vi "Dashboard custom_bartender&global&gripper&camera2-2.vi"() -> ()   [LabVIEW 2017]
uses:
  C:/Users/IMR Lab/Documents/LabVIEW Data/UniversalRobotsSDK_LABView/LabVIEW/Examples/LabVIEW10/UnderAutomation.UniversalRobots.dll
  UnderAutomation.UniversalRobots.dll
  Global 1.vi
panel:
  out "3rd Order":bool
  out "2nd Order":bool
  out "1st Order":bool
  in  "stop":bool
  out "Rx":dbl
  out "Rz":dbl
  out "Ry":dbl
  out "Enabled":bool
  out "Port":i32
  in  "Move to particular posture":bool
  in  "Move to Zero position":bool
  out "Connected":bool
  in  "Robot IP(192.168.112.182)":string
  out "Connect error":errorcluster
  in  "Power on\nRelease brake":bool
  in  "Power off":bool
  in  "Connect":bool
  in  "Send script":bool
  in  "Script to execute":string
  out "Powered on":bool
  out "X":dbl
  out "Y":dbl
  out "Z":dbl
  out "License state":string
  # "e"
  # "movej( get_inverse_kin(p[0.3138, 0.0814, 0.1647, 0.4226, -2.3876, -2.3851]),  a=0.5, v=0.25, t=0, r=0)"
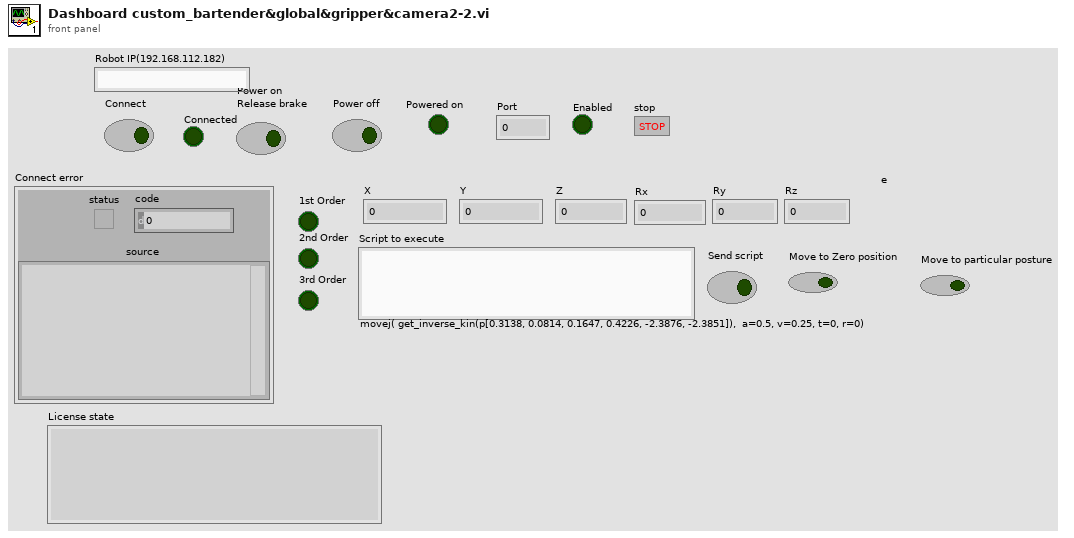
[diagram p1: front panel]
types:
  T1 = enum16{"Standard", "Buffered", "CRLF", "Immediate"}
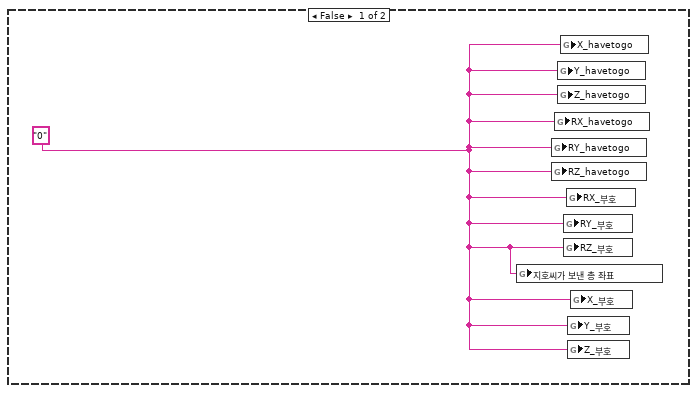
[diagram p2: hidden frame]
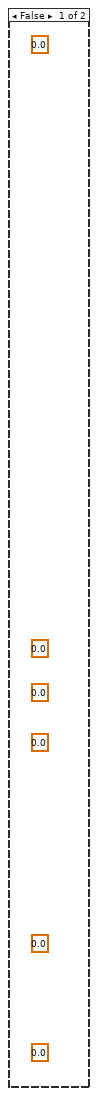
[diagram p3: hidden frame]
diagram:
  w1 = ""
  # "미니콜라 따르는 자세"
  # "술잔 중간지점 가는 자세"
  # "짐빔에서 토닉이동 준비 자세"
  # "술잔 따르는 자세2"
  # "술잔 위로 가는 자세2"
  # "토닉워터 뺴는 자세"
  # "토닉워 들어올리는 자세"
  # "토닉워터 가는 자세"
  # "토닉워터 보는 자세"
  # "짐빔 들어올리는 자세"
  # "짐빔로 가는 자세"
  # "짐빔 보는 자세"
  # "콜라 뺴는 자세"
  # "콜라 들어올리는 자세"
  # "콜라로 가는 자세"
  # "콜라 보는 자세"
  # "술잔 따르는 자세"
  # "술잔 위로 가는 자세"
  # "잭다니엘 들어올리는 자세"
  # "잭다니엘 위치로 가는 자세"
  # "잭다니엘 보는 자세"
  # "1자로 서는 자세"
  # "Example : Display power on status"
  # "Create a UR\ncobot instance"
  # "Show license state"
  # "Register your confidential license key to exit\ntrial period and use this library forever"
  # "Power off when button is clicked"
  # "Power on and release brake when button is clicked"
  # "Get your UR Dashboard interface"
  n1 = global write "Global 1.vi" "TCP 스위치"(FALSE ("TCP 스위치")) -> ()
  n2 = global write "Global 1.vi" "미니콜라 따르는 자세"("movej([-0.0902,-1.8120,-1.9241,-3.5769,6.2827,8.4658], a=0.5, v=0.25, t=0, r=0)") -> ()
  n3 = global write "Global 1.vi" "잭다니엘 들어올리는 자세"("movej([0.8116,-2.0223,-1.2828,-3.0107,4.3284,5.9341], a=0.5, v=0.25, t=0, r=0)") -> ()
  n4 = global write "Global 1.vi" "짐빔 토닉 이동 준비자세"("movej([-0.5421,-0.8131,0.8439,-0.0538,2.5052,5.9032], a=0.5, v=0.25, t=0, r=0)") -> ()
  n5 = global write "Global 1.vi" "토닉 빼는 자세"("movej([-0.5277,-1.5104,1.5889,-0.0548,2.5728,5.9025], a=0.5, v=0.25, t=0, r=0)") -> ()
  n6 = global write "Global 1.vi" "잭다닐 위치로 가는 자세"("movej([0.8116,-2.3119,-1.606,-2.3958,4.3284,5.9341], a=0.5, v=0.25, t=0, r=0)") -> ()
  n7 = global write "Global 1.vi" "토닉 드는 자세"("movej([-1.0311,-1.1460,1.5830,-0.4348,2.0708,5.9048], a=0.5, v=0.25, t=0, r=0)") -> ()
  n8 = global write "Global 1.vi" "토닉 보는 자세"("movej([-0.4690,-1.1292,2.1508,-1.0119,2.6124,5.9032], a=0.5, v=0.25, t=0, r=0)") -> ()
  n9 = global write "Global 1.vi" "술잔 위로 가는 자세 2"("movej([0.0485,-1.6015,2.5780,-1.0382,-0.0520,5.3649], a=0.5, v=0.25, t=0, r=0)") -> ()
  n10 = global write "Global 1.vi" "1자로 서는 자세"("movej([3.1412,-1.5708,0,-1.5708,3.1412,5.8904], a=0.5, v=0.25, t=0, r=0)") -> ()
  n11 = global write "Global 1.vi" "짐빔 들어올리는 자세"("movej([-0.5421,-0.8131,0.8439,-0.0538,2.5052,5.9032], a=0.5, v=0.25, t=0, r=0)") -> ()
  n12 = global write "Global 1.vi" "술잔 위로 가는 자세"("movej([-0.0903,-2.0548,-2.0169,-3.3289,6.2826,7.4091], a=0.5, v=0.25, t=0, r=0)") -> ()
  n13 = global write "Global 1.vi" "토닉 가는자세"("movej([-0.9924,-0.8742,1.7459,-0.8837,2.0958,5.9048], a=0.5, v=0.25, t=0, r=0)") -> ()
  n14 = global write "Global 1.vi" "잭다니엘 보는 자세"("movej([0,-2.2170,-1.4226,-2.2842,3.1412,6.2832], a=0.5, v=0.25, t=0, r=0)") -> ()
  n15 = global write "Global 1.vi" "짐빔 위치로 가는 자세"("movej([-0.5436,-0.4519,0.8428,-0.3534,2.6134,5.9032], a=0.5, v=0.25, t=0, r=0)") -> ()
  n16 = global write "Global 1.vi" "콜라 보는 자세"("movej([0,-1.8110,-2.1684,-2.3033,3.1543,5.9213], a=0.5, v=0.25, t=0, r=0)") -> ()
  n17 = global write "Global 1.vi" "콜라로 가는자세"("movej([1.2020,-2.166,-1.9385,-2.1863,4.3172,5.9210], a=0.5, v=0.25, t=0, r=0)") -> ()
  n18 = global write "Global 1.vi" "콜라 빼는 자세"("movej([0.8789,-1.5237,-2.1070,-2.6679, 3.9917,5.9085], a=0.5, v=0.25, t=0, r=0)") -> ()
  n19 = global write "Global 1.vi" "콜라 드는 자세"("movej([1.2020,-1.8452,-1.7403,-2.7082,4.3162,5.9158], a=0.5, v=0.25, t=0, r=0)") -> ()
  n20 = global write "Global 1.vi" "술 따르는 자세 2"("movej([0.0412,-1.9708,2.4700,-1.0157,-0.0618,4.8998], a=0.5, v=0.25, t=0, r=0)") -> ()
  n21 = global write "Global 1.vi" "잭다니엘 카메라 값"(w1) -> ()
  n22 = global write "Global 1.vi" "술 따르는 자세"("movej([-0.0902,-1.9024,-1.9241,-3.5769,6.2827,8.4692], a=0.5, v=0.25, t=0, r=0)") -> ()
  n23 = global write "Global 1.vi" "짐빔 보는 자세"("movej([-0.0364,-0.6154,0.9421,-0.3291,3.1047,5.9020], a=0.5, v=0.25, t=0, r=0)") -> ()
  n24 = global write "Global 1.vi" "콜라 카메라 값"(w1) -> ()
  n25 = global write "Global 1.vi" "토닉 카메라 값"(w1) -> ()
  n26 = global write "Global 1.vi" "짐빔 카메라 값"(w1) -> ()
  n27 = constructor class="UR"() -> (reference out=w27:refnum<k24>)  [unwired: 3 in, 2 out]
  n28 = global write "Global 1.vi" "술잔 중간지점"("movej([-0.2173,-1.9485,-1.6874,-3.9352,6.2671,7.2276], a=0.5, v=0.25, t=0, r=0)") -> ()
  n29 = while {
    tunnel: w27 -> [w33]
    stop <- FALSE stop-if-true
    # "Connect to the robot when button is pressed"
    # "Show if primary interface is connected"
    # "Get your UR primary interface"
    n30 = property class="UR"(reference=w33) -> ("PrimaryInterface"=w36:refnum<k24>)  [unwired: 1 in, 2 out]
    n31 = Wait (ms)(milliseconds to wait=u32 50) -> ()  [unwired: 1 out]
    n32 = property class="PrimaryInterfaceClientInternal"(reference=w36) -> ("Connected"=w35:bool)  [unwired: 1 in, 2 out]
    "Connected" <- w35
    n33 = case shown="True" "Connect" {
      tunnel: w33 -> [_ w1119]
      frame False {
      }
      frame True {
        n34 = flat-sequence {
          tunnel: w1119 -> [w1121]
          frame #0 {
            n35 = invoke class="UR" method="Connect"(reference=w1121, "ip"="Robot IP(192.168.112.182)") -> (error out=→"Connect error":errorcluster)  [unwired: 2 in, 3 out]
          }
        }
      }
    }
    n36 = case shown="True" w35 {
      tunnel: w36 -> [_ w49]
      frame False {
        (unwired) 0.0 ("Rx")
        (unwired) 0.0 ("Rz")
        (unwired) 0.0 ("Ry")
        (unwired) 0.0 ("Z")
        (unwired) 0.0 ("X")
        (unwired) 0.0 ("Y")
      }
      frame True {
        # "Send URScript when button pressed"
        # "Example : Display current cartesian pose"
        n37 = property class="PrimaryInterfaceClientInternal"(reference=w49) -> ("Script"=w50:refnum<k24>)  [unwired: 1 in, 2 out]
        n38 = global read "Global 1.vi" "2nd Order"() -> (w53:bool)
        "2nd Order" <- w53
        n39 = global read "Global 1.vi" "3rd Order"() -> (w52:bool)
        "3rd Order" <- w52
        n40 = global read "Global 1.vi" "1st Order"() -> (w54:bool)
        "1st Order" <- w54
        n41 = Build Array(w54, w53, w52) -> (w55:bool[])
        n42 = Boolean Array To Number(Boolean array=w55) -> (number=w51:u32)
        n43 = case shown="100" w51 {
          tunnel: w50 -> [_ w106 w433 _ w763 _ _ _]
          frame 0, Default {
          }
          frame 1 {
            # "잭다 : 콜라 = 1 : 3"
            # "1st order"
            n44 = flat-sequence {
              tunnel: w106 -> [w110]
              tunnel: [w109] -> w105
              tunnel: w105 -> [w114]
              tunnel: [w112] -> w99
              tunnel: w99 -> [w117]
              tunnel: [w117] -> w97
              tunnel: w97 -> [w120]
              tunnel: [w120] -> w75
              tunnel: w75 -> [w124]
              tunnel: [w124] -> w72
              tunnel: w72 -> [w131]
              tunnel: [w131] -> w71
              tunnel: w71 -> [w207]
              tunnel: [w207] -> w74
              tunnel: w74 -> [w210]
              tunnel: [w210] -> w73
              tunnel: w73 -> [w214]
              tunnel: [w211] -> w98
              tunnel: w98 -> [w217]
              tunnel: [w217] -> w96
              tunnel: w96 -> [w220]
              tunnel: [w220] -> w95
              tunnel: w95 -> [w222]
              tunnel: [w221] -> w83
              tunnel: w83 -> [w226]
              tunnel: [w225] -> w82
              tunnel: w82 -> [w230]
              tunnel: [w229] -> w104
              tunnel: w104 -> [w235]
              tunnel: [w233] -> w103
              tunnel: w103 -> [w238]
              tunnel: [w237] -> w81
              tunnel: w81 -> [w242]
              tunnel: [w241] -> w80
              tunnel: [w245] -> w70
              tunnel: w80 -> [w247]
              tunnel: [w249] -> w94
              tunnel: w70 -> [w250]
              tunnel: w94 -> [w255]
              tunnel: [w255] -> w93
              tunnel: w93 -> [w258]
              tunnel: [w258] -> w92
              tunnel: w92 -> [w260]
              tunnel: [w259] -> w68
              tunnel: w68 -> [w266]
              tunnel: [w266] -> w67
              tunnel: w67 -> [w273]
              tunnel: [w273] -> w66
              tunnel: w66 -> [w349]
              tunnel: [w349] -> w65
              tunnel: w65 -> [w352]
              tunnel: [w352] -> w64
              tunnel: [w353] -> w91
              tunnel: w64 -> [w354]
              tunnel: w91 -> [w359]
              tunnel: [w359] -> w90
              tunnel: w90 -> [w362]
              tunnel: [w362] -> w69
              tunnel: [w363] -> w89
              tunnel: w69 -> [w364]
              tunnel: w89 -> [w368]
              tunnel: [w367] -> w79
              tunnel: w79 -> [w372]
              tunnel: [w371] -> w78
              tunnel: w78 -> [w376]
              tunnel: [w375] -> w102
              tunnel: w102 -> [w380]
              tunnel: [w379] -> w101
              tunnel: w101 -> [w384]
              tunnel: [w383] -> w77
              tunnel: w77 -> [w388]
              tunnel: [w387] -> w76
              tunnel: w76 -> [w392]
              tunnel: [w391] -> w88
              tunnel: w88 -> [w396]
              tunnel: [w395] -> w100
              tunnel: w100 -> [w400]
              tunnel: [w399] -> w86
              tunnel: [w403] -> w87
              tunnel: w86 -> [w403]
              tunnel: [w406] -> w85
              tunnel: w87 -> [w406]
              tunnel: w85 -> [w410]
              tunnel: [w409] -> w84
              tunnel: w84 -> [w413]
              frame #0 {
                # "초기자세"
                n45 = global read "Global 1.vi" "1자로 서는 자세"() -> (w108:string)
                n46 = invoke class="PrimaryInterfaceScript" method="Send"(reference=w110, "script"=w108) -> (reference out=w109:refnum<k24>)  [unwired: 2 in, 3 out]
                n47 = Wait (ms)(milliseconds to wait=u32 15000) -> ()  [unwired: 1 out]
              }
              frame #1 {
                # "잭다니엘 보기"
                n48 = global read "Global 1.vi" "잭다니엘 보는 자세"() -> (w113:string)
                n49 = invoke class="PrimaryInterfaceScript" method="Send"(reference=w114, "script"=w113) -> (reference out=w112:refnum<k24>)  [unwired: 2 in, 3 out]
                n50 = Wait (ms)(milliseconds to wait=u32 15000) -> ()  [unwired: 1 out]
              }
              frame #2 {
                # "그리퍼 열기"
                n51 = global write "Global 1.vi" "그리퍼 열림"(TRUE ("그리퍼 열림")) -> ()
                n52 = Wait (ms)(milliseconds to wait=u32 300) -> ()  [unwired: 1 out]
              }
              frame #3 {
                n53 = global write "Global 1.vi" "그리퍼 열림"(FALSE ("그리퍼 열림")) -> ()
                n54 = Wait (ms)(milliseconds to wait=u32 300) -> ()  [unwired: 1 out]
              }
              frame #4 {
                # "tcp 키는 스위치 보단\n파이썬한테 \n값 보내달라하는\n요청 보내는 걸로 \n바꾸기"
                n55 = global write "Global 1.vi" "몇번 병을 볼것인가"("0" ("몇번 병을 볼것인가")) -> ()
                n56 = global write "Global 1.vi" "TCP 스위치"(TRUE ("그리퍼 열림")) -> ()
                n57 = Wait Until Next ms Multiple(millisecond multiple=u32 500 ("milliseconds to wait")) -> ()  [unwired: 1 out]
              }
              frame #5 {
                n58 = global read "Global 1.vi" "X_부호"() -> (w127:string)
                n59 = global read "Global 1.vi" "Z_부호"() -> (w125:string)
                n60 = global read "Global 1.vi" "Y_부호"() -> (w126:string)
                n61 = case shown="\"1\"" w125 {
                  frame "False", Default {
                  }
                  frame "True" {
                  }
                  frame "2" {
                  }
                  frame "1" {
                    n62 = global read "Global 1.vi" "Z_havetogo"() -> (w133:string)
                    n63 = Decimal String To Number(string=w133) -> (number=w136:i32)  [unwired: 2 in, 1 out]
                    n64 = To Double Precision Float(number=w136) -> (double precision float=w135:dbl)
                    n65 = Format Into String(format string="-%f", w135) -> (resulting string=w132:string)  [unwired: 2 in, 1 out]
                    n66 = global write "Global 1.vi" "Z_havetogo"(w132) -> ()
                  }
                }
                n67 = case shown="\"1\"" w126 {
                  frame "False", Default {
                  }
                  frame "True" {
                  }
                  frame "2" {
                  }
                  frame "1" {
                    n68 = global read "Global 1.vi" "Y_havetogo"() -> (w138:string)
                    n69 = Decimal String To Number(string=w138) -> (number=w141:i32)  [unwired: 2 in, 1 out]
                    n70 = To Double Precision Float(number=w141) -> (double precision float=w139:dbl)
                    n71 = Format Into String(format string="-%f", w139) -> (resulting string=w137:string)  [unwired: 2 in, 1 out]
                    n72 = global write "Global 1.vi" "Y_havetogo"(w137) -> ()
                  }
                }
                n73 = case shown="\"1\"" w127 {
                  frame "False", Default {
                  }
                  frame "True" {
                  }
                  frame "2" {
                  }
                  frame "1" {
                    n74 = global read "Global 1.vi" "X_havetogo"() -> (w143:string)
                    n75 = Decimal String To Number(string=w143) -> (number=w146:i32)  [unwired: 2 in, 1 out]
                    n76 = To Double Precision Float(number=w146) -> (double precision float=w145:dbl)
                    n77 = Format Into String(format string="-%f", w145) -> (resulting string=w142:string)  [unwired: 2 in, 1 out]
                    n78 = global write "Global 1.vi" "X_havetogo"(w142) -> ()
                  }
                }
                n79 = global read "Global 1.vi" "RX_부호"() -> (w130:string)
                n80 = global read "Global 1.vi" "RZ_부호"() -> (w128:string)
                n81 = global read "Global 1.vi" "RY_부호"() -> (w129:string)
                n82 = case shown="\"1\"" w128 {
                  frame "False", Default {
                  }
                  frame "True" {
                  }
                  frame "2" {
                  }
                  frame "1" {
                    n83 = global read "Global 1.vi" "RZ_havetogo"() -> (w148:string)
                    n84 = Decimal String To Number(string=w148) -> (number=w151:i32)  [unwired: 2 in, 1 out]
                    n85 = To Double Precision Float(number=w151) -> (double precision float=w150:dbl)
                    n86 = Format Into String(format string="-%f", w150) -> (resulting string=w147:string)  [unwired: 2 in, 1 out]
                    n87 = global write "Global 1.vi" "RZ_havetogo"(w147) -> ()
                  }
                }
                n88 = case shown="\"1\"" w129 {
                  frame "False", Default {
                  }
                  frame "True" {
                  }
                  frame "2" {
                  }
                  frame "1" {
                    n89 = global read "Global 1.vi" "RY_havetogo"() -> (w153:string)
                    n90 = Decimal String To Number(string=w153) -> (number=w156:i32)  [unwired: 2 in, 1 out]
                    n91 = To Double Precision Float(number=w156) -> (double precision float=w154:dbl)
                    n92 = Format Into String(format string="-%f", w154) -> (resulting string=w152:string)  [unwired: 2 in, 1 out]
                    n93 = global write "Global 1.vi" "RY_havetogo"(w152) -> ()
                  }
                }
                n94 = case shown="\"1\"" w130 {
                  frame "False", Default {
                  }
                  frame "True" {
                  }
                  frame "2" {
                  }
                  frame "1" {
                    n95 = global read "Global 1.vi" "RX_havetogo"() -> (w158:string)
                    n96 = Decimal String To Number(string=w158) -> (number=w161:i32)  [unwired: 2 in, 1 out]
                    n97 = To Double Precision Float(number=w161) -> (double precision float=w160:dbl)
                    n98 = Format Into String(format string="-%f", w160) -> (resulting string=w157:string)  [unwired: 2 in, 1 out]
                    n99 = global write "Global 1.vi" "RX_havetogo"(w157) -> ()
                  }
                }
              }
              frame #6 {
                n100 = global read "Global 1.vi" "X_havetogo"() -> (w173:string)
                n101 = global read "Global 1.vi" "Y_havetogo"() -> (w172:string)
                n102 = global read "Global 1.vi" "Z_havetogo"() -> (w171:string)
                n103 = global read "Global 1.vi" "RX_havetogo"() -> (w170:string)
                n104 = global read "Global 1.vi" "RY_havetogo"() -> (w169:string)
                n105 = global read "Global 1.vi" "RZ_havetogo"() -> (w168:string)
                n106 = Decimal String To Number(string=w171) -> (number=w197:i32)  [unwired: 2 in, 1 out]
                n107 = Decimal String To Number(string=w173) -> (number=w203:i32)  [unwired: 2 in, 1 out]
                n108 = Decimal String To Number(string=w172) -> (number=w200:i32)  [unwired: 2 in, 1 out]
                n109 = Decimal String To Number(string=w170) -> (number=w194:i32)  [unwired: 2 in, 1 out]
                n110 = Decimal String To Number(string=w169) -> (number=w191:i32)  [unwired: 2 in, 1 out]
                n111 = Decimal String To Number(string=w168) -> (number=w188:i32)  [unwired: 2 in, 1 out]
                n112 = To Double Precision Float(number=w197) -> (double precision float=w199:dbl)
                n113 = To Double Precision Float(number=w203) -> (double precision float=w205:dbl)
                n114 = To Double Precision Float(number=w200) -> (double precision float=w202:dbl)
                n115 = To Double Precision Float(number=w194) -> (double precision float=w196:dbl)
                n116 = To Double Precision Float(number=w191) -> (double precision float=w193:dbl)
                n117 = Multiply(x=w205, y=0.001) -> (x*y=w187:dbl)
                n118 = Multiply(x=w199, y=0.001) -> (x*y=w183:dbl)
                n119 = Multiply(x=w202, y=0.001) -> (x*y=w185:dbl)
                n120 = Multiply(x=w196, y=0.001) -> (x*y=w181:dbl)
                n121 = global read "Global 1.vi" "x"() -> (w167:dbl)
                n122 = Multiply(x=w193, y=0.001) -> (x*y=w179:dbl)
                n123 = global read "Global 1.vi" "y"() -> (w166:dbl)
                n124 = global read "Global 1.vi" "rx"() -> (w164:dbl)
                n125 = global read "Global 1.vi" "z"() -> (w165:dbl)
                n126 = To Double Precision Float(number=w188) -> (double precision float=w190:dbl)
                n127 = Add(x=w167, y=w187) -> (x+y=w186:dbl)
                n128 = Multiply(x=w190, y=0.001) -> (x*y=w177:dbl)
                n129 = Add(x=w183, y=w165) -> (x+y=w182:dbl)
                n130 = Add(x=w185, y=w166) -> (x+y=w184:dbl)
                n131 = global read "Global 1.vi" "ry"() -> (w162:dbl)
                n132 = global read "Global 1.vi" "rz"() -> (w163:dbl)
                n133 = Add(x=w181, y=w164) -> (x+y=w180:dbl)
                n134 = Add(x=w179, y=w162) -> (x+y=w178:dbl)
                n135 = Add(x=w177, y=w163) -> (x+y=w176:dbl)
                n136 = Format Into String(format string="movej( get_inverse_kin(p[%f, %f, %f, %f, %f, %f]), a= 0.5, v=0.25, t=0, r=0)", w186, w184, w182, w180, w178, w176) -> (resulting string=w174:string)  [unwired: 2 in, 1 out]
                n137 = global write "Global 1.vi" "잭다니엘 카메라 값"(w174) -> ()
                n138 = Wait (ms)(milliseconds to wait=u32 300) -> ()  [unwired: 1 out]
              }
              frame #7 {
                n139 = global write "Global 1.vi" "TCP 스위치"(FALSE ("그리퍼 열림")) -> ()
                n140 = Wait Until Next ms Multiple(millisecond multiple=u32 300 ("milliseconds to wait")) -> ()  [unwired: 1 out]
              }
              frame #8 {
                # "잭다니엘 위치로 가기"
                n141 = global read "Global 1.vi" "잭다니엘 카메라 값"() -> (w213:string)
                n142 = invoke class="PrimaryInterfaceScript" method="Send"(reference=w214, "script"=w213) -> (reference out=w211:refnum<k24>)  [unwired: 2 in, 3 out]
                n143 = Wait (ms)(milliseconds to wait=u32 7000) -> ()  [unwired: 1 out]
              }
              frame #9 {
                # "그리퍼 닫기"
                n144 = global write "Global 1.vi" "그리퍼 닫힘"(TRUE ("그리퍼 열림")) -> ()
                n145 = Wait (ms)(milliseconds to wait=u32 300) -> ()  [unwired: 1 out]
              }
              frame #10 {
                n146 = global write "Global 1.vi" "그리퍼 닫힘"(FALSE ("그리퍼 열림")) -> ()
                n147 = Wait (ms)(milliseconds to wait=u32 3000) -> ()  [unwired: 1 out]
              }
              frame #11 {
                # "잭다니엘 들기"
                n148 = global read "Global 1.vi" "잭다니엘 들어올리는 자세"() -> (w224:string)
                n149 = invoke class="PrimaryInterfaceScript" method="Send"(reference=w222, "script"=w224) -> (reference out=w221:refnum<k24>)  [unwired: 2 in, 3 out]
                n150 = Wait (ms)(milliseconds to wait=u32 5000) -> ()  [unwired: 1 out]
              }
              frame #12 {
                # "술잔 중간지점으로 이동"
                n151 = global read "Global 1.vi" "술잔 중간지점"() -> (w227:string)
                n152 = invoke class="PrimaryInterfaceScript" method="Send"(reference=w226, "script"=w227) -> (reference out=w225:refnum<k24>)  [unwired: 2 in, 3 out]
                n153 = Wait (ms)(milliseconds to wait=u32 15000) -> ()  [unwired: 1 out]
              }
              frame #13 {
                # "술잔 쪽으로 이동"
                n154 = global read "Global 1.vi" "술잔 위로 가는 자세"() -> (w231:string)
                n155 = invoke class="PrimaryInterfaceScript" method="Send"(reference=w230, "script"=w231) -> (reference out=w229:refnum<k24>)  [unwired: 2 in, 3 out]
                n156 = Wait (ms)(milliseconds to wait=u32 5000) -> ()  [unwired: 1 out]
              }
              frame #14 {
                # "술따르기"
                n157 = global read "Global 1.vi" "술 따르는 자세"() -> (w234:string)
                n158 = invoke class="PrimaryInterfaceScript" method="Send"(reference=w235, "script"=w234) -> (reference out=w233:refnum<k24>)  [unwired: 2 in, 3 out]
                n159 = Wait (ms)(milliseconds to wait=u32 9000) -> ()  [unwired: 1 out]
              }
              frame #15 {
                # "술따르기 중단"
                n160 = global read "Global 1.vi" "술잔 위로 가는 자세"() -> (w239:string)
                n161 = invoke class="PrimaryInterfaceScript" method="Send"(reference=w238, "script"=w239) -> (reference out=w237:refnum<k24>)  [unwired: 2 in, 3 out]
                n162 = Wait (ms)(milliseconds to wait=u32 4000) -> ()  [unwired: 1 out]
              }
              frame #16 {
                # "술잔 중간지점으로 이동"
                n163 = global read "Global 1.vi" "술잔 중간지점"() -> (w243:string)
                n164 = invoke class="PrimaryInterfaceScript" method="Send"(reference=w242, "script"=w243) -> (reference out=w241:refnum<k24>)  [unwired: 2 in, 3 out]
                n165 = Wait (ms)(milliseconds to wait=u32 7000) -> ()  [unwired: 1 out]
              }
              frame #17 {
                # "잭다니엘 들었던 곳으로"
                n166 = global read "Global 1.vi" "잭다니엘 들어올리는 자세"() -> (w246:string)
                n167 = invoke class="PrimaryInterfaceScript" method="Send"(reference=w247, "script"=w246) -> (reference out=w245:refnum<k24>)  [unwired: 2 in, 3 out]
                n168 = Wait (ms)(milliseconds to wait=u32 10000) -> ()  [unwired: 1 out]
              }
              frame #18 {
                # "잭다니엘 내려놓기"
                n169 = global read "Global 1.vi" "잭다닐 위치로 가는 자세"() -> (w252:string)
                n170 = invoke class="PrimaryInterfaceScript" method="Send"(reference=w250, "script"=w252) -> (reference out=w249:refnum<k24>)  [unwired: 2 in, 3 out]
                n171 = Wait (ms)(milliseconds to wait=u32 5000) -> ()  [unwired: 1 out]
              }
              frame #19 {
                # "그리퍼 열기"
                n172 = global write "Global 1.vi" "그리퍼 열림"(TRUE ("그리퍼 열림")) -> ()
                n173 = Wait (ms)(milliseconds to wait=u32 300) -> ()  [unwired: 1 out]
              }
              frame #20 {
                n174 = global write "Global 1.vi" "그리퍼 열림"(FALSE ("그리퍼 열림")) -> ()
                n175 = Wait (ms)(milliseconds to wait=u32 3000) -> ()  [unwired: 1 out]
              }
              frame #21 {
                # "콜라보러가기"
                n176 = global read "Global 1.vi" "콜라 보는 자세"() -> (w262:string)
                n177 = invoke class="PrimaryInterfaceScript" method="Send"(reference=w260, "script"=w262) -> (reference out=w259:refnum<k24>)  [unwired: 2 in, 3 out]
                n178 = Wait (ms)(milliseconds to wait=u32 8000) -> ()  [unwired: 1 out]
              }
              frame #22 {
                # "tcp 키는 스위치 보단\n파이썬한테 \n값 보내달라하는\n요청 보내는 걸로 \n바꾸기"
                n179 = global write "Global 1.vi" "몇번 병을 볼것인가"("1" ("몇번 병을 볼것인가")) -> ()
                n180 = global write "Global 1.vi" "TCP 스위치"(TRUE ("그리퍼 열림")) -> ()
                n181 = Wait Until Next ms Multiple(millisecond multiple=u32 500 ("milliseconds to wait")) -> ()  [unwired: 1 out]
              }
              frame #23 {
                n182 = global read "Global 1.vi" "X_부호"() -> (w269:string)
                n183 = global read "Global 1.vi" "Z_부호"() -> (w267:string)
                n184 = global read "Global 1.vi" "Y_부호"() -> (w268:string)
                n185 = case shown="\"1\"" w267 {
                  frame "False", Default {
                  }
                  frame "True" {
                  }
                  frame "2" {
                  }
                  frame "1" {
                    n186 = global read "Global 1.vi" "Z_havetogo"() -> (w275:string)
                    n187 = Decimal String To Number(string=w275) -> (number=w278:i32)  [unwired: 2 in, 1 out]
                    n188 = To Double Precision Float(number=w278) -> (double precision float=w277:dbl)
                    n189 = Format Into String(format string="-%f", w277) -> (resulting string=w274:string)  [unwired: 2 in, 1 out]
                    n190 = global write "Global 1.vi" "Z_havetogo"(w274) -> ()
                  }
                }
                n191 = case shown="\"1\"" w268 {
                  frame "False", Default {
                  }
                  frame "True" {
                  }
                  frame "2" {
                  }
                  frame "1" {
                    n192 = global read "Global 1.vi" "Y_havetogo"() -> (w280:string)
                    n193 = Decimal String To Number(string=w280) -> (number=w283:i32)  [unwired: 2 in, 1 out]
                    n194 = To Double Precision Float(number=w283) -> (double precision float=w281:dbl)
                    n195 = Format Into String(format string="-%f", w281) -> (resulting string=w279:string)  [unwired: 2 in, 1 out]
                    n196 = global write "Global 1.vi" "Y_havetogo"(w279) -> ()
                  }
                }
                n197 = case shown="\"1\"" w269 {
                  frame "False", Default {
                  }
                  frame "True" {
                  }
                  frame "2" {
                  }
                  frame "1" {
                    n198 = global read "Global 1.vi" "X_havetogo"() -> (w285:string)
                    n199 = Decimal String To Number(string=w285) -> (number=w288:i32)  [unwired: 2 in, 1 out]
                    n200 = To Double Precision Float(number=w288) -> (double precision float=w287:dbl)
                    n201 = Format Into String(format string="-%f", w287) -> (resulting string=w284:string)  [unwired: 2 in, 1 out]
                    n202 = global write "Global 1.vi" "X_havetogo"(w284) -> ()
                  }
                }
                n203 = global read "Global 1.vi" "RX_부호"() -> (w272:string)
                n204 = global read "Global 1.vi" "RZ_부호"() -> (w270:string)
                n205 = global read "Global 1.vi" "RY_부호"() -> (w271:string)
                n206 = case shown="\"1\"" w270 {
                  frame "False", Default {
                  }
                  frame "True" {
                  }
                  frame "2" {
                  }
                  frame "1" {
                    n207 = global read "Global 1.vi" "RZ_havetogo"() -> (w290:string)
                    n208 = Decimal String To Number(string=w290) -> (number=w293:i32)  [unwired: 2 in, 1 out]
                    n209 = To Double Precision Float(number=w293) -> (double precision float=w292:dbl)
                    n210 = Format Into String(format string="-%f", w292) -> (resulting string=w289:string)  [unwired: 2 in, 1 out]
                    n211 = global write "Global 1.vi" "RZ_havetogo"(w289) -> ()
                  }
                }
                n212 = case shown="\"1\"" w271 {
                  frame "False", Default {
                  }
                  frame "True" {
                  }
                  frame "2" {
                  }
                  frame "1" {
                    n213 = global read "Global 1.vi" "RY_havetogo"() -> (w295:string)
                    n214 = Decimal String To Number(string=w295) -> (number=w298:i32)  [unwired: 2 in, 1 out]
                    n215 = To Double Precision Float(number=w298) -> (double precision float=w296:dbl)
                    n216 = Format Into String(format string="-%f", w296) -> (resulting string=w294:string)  [unwired: 2 in, 1 out]
                    n217 = global write "Global 1.vi" "RY_havetogo"(w294) -> ()
                  }
                }
                n218 = case shown="\"1\"" w272 {
                  frame "False", Default {
                  }
                  frame "True" {
                  }
                  frame "2" {
                  }
                  frame "1" {
                    n219 = global read "Global 1.vi" "RX_havetogo"() -> (w300:string)
                    n220 = Decimal String To Number(string=w300) -> (number=w303:i32)  [unwired: 2 in, 1 out]
                    n221 = To Double Precision Float(number=w303) -> (double precision float=w302:dbl)
                    n222 = Format Into String(format string="-%f", w302) -> (resulting string=w299:string)  [unwired: 2 in, 1 out]
                    n223 = global write "Global 1.vi" "RX_havetogo"(w299) -> ()
                  }
                }
              }
              frame #24 {
                n224 = global read "Global 1.vi" "X_havetogo"() -> (w315:string)
                n225 = global read "Global 1.vi" "Y_havetogo"() -> (w314:string)
                n226 = global read "Global 1.vi" "Z_havetogo"() -> (w313:string)
                n227 = global read "Global 1.vi" "RX_havetogo"() -> (w312:string)
                n228 = global read "Global 1.vi" "RY_havetogo"() -> (w311:string)
                n229 = global read "Global 1.vi" "RZ_havetogo"() -> (w310:string)
                n230 = Decimal String To Number(string=w313) -> (number=w339:i32)  [unwired: 2 in, 1 out]
                n231 = Decimal String To Number(string=w315) -> (number=w345:i32)  [unwired: 2 in, 1 out]
                n232 = Decimal String To Number(string=w314) -> (number=w342:i32)  [unwired: 2 in, 1 out]
                n233 = Decimal String To Number(string=w312) -> (number=w336:i32)  [unwired: 2 in, 1 out]
                n234 = Decimal String To Number(string=w311) -> (number=w333:i32)  [unwired: 2 in, 1 out]
                n235 = Decimal String To Number(string=w310) -> (number=w330:i32)  [unwired: 2 in, 1 out]
                n236 = To Double Precision Float(number=w339) -> (double precision float=w341:dbl)
                n237 = To Double Precision Float(number=w345) -> (double precision float=w347:dbl)
                n238 = To Double Precision Float(number=w342) -> (double precision float=w344:dbl)
                n239 = To Double Precision Float(number=w336) -> (double precision float=w338:dbl)
                n240 = To Double Precision Float(number=w333) -> (double precision float=w335:dbl)
                n241 = Multiply(x=w347, y=0.001) -> (x*y=w329:dbl)
                n242 = Multiply(x=w341, y=0.001) -> (x*y=w325:dbl)
                n243 = Multiply(x=w344, y=0.001) -> (x*y=w327:dbl)
                n244 = Multiply(x=w338, y=0.001) -> (x*y=w323:dbl)
                n245 = global read "Global 1.vi" "x"() -> (w309:dbl)
                n246 = Multiply(x=w335, y=0.001) -> (x*y=w321:dbl)
                n247 = global read "Global 1.vi" "y"() -> (w308:dbl)
                n248 = global read "Global 1.vi" "rx"() -> (w306:dbl)
                n249 = global read "Global 1.vi" "z"() -> (w307:dbl)
                n250 = To Double Precision Float(number=w330) -> (double precision float=w332:dbl)
                n251 = Add(x=w309, y=w329) -> (x+y=w328:dbl)
                n252 = Multiply(x=w332, y=0.001) -> (x*y=w319:dbl)
                n253 = Add(x=w325, y=w307) -> (x+y=w324:dbl)
                n254 = Add(x=w327, y=w308) -> (x+y=w326:dbl)
                n255 = global read "Global 1.vi" "ry"() -> (w304:dbl)
                n256 = global read "Global 1.vi" "rz"() -> (w305:dbl)
                n257 = Add(x=w323, y=w306) -> (x+y=w322:dbl)
                n258 = Add(x=w321, y=w304) -> (x+y=w320:dbl)
                n259 = Add(x=w319, y=w305) -> (x+y=w318:dbl)
                n260 = Format Into String(format string="movej( get_inverse_kin(p[%f, %f, %f, %f, %f, %f]), a= 0.5, v=0.25, t=0, r=0)", w328, w326, w324, w322, w320, w318) -> (resulting string=w316:string)  [unwired: 2 in, 1 out]
                n261 = global write "Global 1.vi" "콜라 카메라 값"(w316) -> ()
                n262 = Wait (ms)(milliseconds to wait=u32 300) -> ()  [unwired: 1 out]
              }
              frame #25 {
                n263 = global write "Global 1.vi" "TCP 스위치"(FALSE ("그리퍼 열림")) -> ()
                n264 = Wait Until Next ms Multiple(millisecond multiple=u32 300 ("milliseconds to wait")) -> ()  [unwired: 1 out]
              }
              frame #26 {
                # "콜라 들러가기"
                n265 = global read "Global 1.vi" "콜라 카메라 값"() -> (w356:string)
                n266 = invoke class="PrimaryInterfaceScript" method="Send"(reference=w354, "script"=w356) -> (reference out=w353:refnum<k24>)  [unwired: 2 in, 3 out]
                n267 = Wait (ms)(milliseconds to wait=u32 8000) -> ()  [unwired: 1 out]
              }
              frame #27 {
                n268 = global write "Global 1.vi" "그리퍼 닫힘"(TRUE ("그리퍼 열림")) -> ()
                n269 = Wait (ms)(milliseconds to wait=u32 300) -> ()  [unwired: 1 out]
              }
              frame #28 {
                n270 = global write "Global 1.vi" "그리퍼 닫힘"(FALSE ("그리퍼 열림")) -> ()
                n271 = Wait (ms)(milliseconds to wait=u32 3000) -> ()  [unwired: 1 out]
              }
              frame #29 {
                # "콜라 들어올리기"
                n272 = global read "Global 1.vi" "콜라 드는 자세"() -> (w366:string)
                n273 = invoke class="PrimaryInterfaceScript" method="Send"(reference=w364, "script"=w366) -> (reference out=w363:refnum<k24>)  [unwired: 2 in, 3 out]
                n274 = Wait (ms)(milliseconds to wait=u32 5000) -> ()  [unwired: 1 out]
              }
              frame #30 {
                # "콜라 살짝 빼기"
                n275 = global read "Global 1.vi" "콜라 빼는 자세"() -> (w370:string)
                n276 = invoke class="PrimaryInterfaceScript" method="Send"(reference=w368, "script"=w370) -> (reference out=w367:refnum<k24>)  [unwired: 2 in, 3 out]
                n277 = Wait (ms)(milliseconds to wait=u32 5000) -> ()  [unwired: 1 out]
              }
              frame #31 {
                # "술잔 중간지점으로 이동"
                n278 = global read "Global 1.vi" "술잔 중간지점"() -> (w373:string)
                n279 = invoke class="PrimaryInterfaceScript" method="Send"(reference=w372, "script"=w373) -> (reference out=w371:refnum<k24>)  [unwired: 2 in, 3 out]
                n280 = Wait (ms)(milliseconds to wait=u32 15000) -> ()  [unwired: 1 out]
              }
              frame #32 {
                # "술잔으로 이동"
                n281 = global read "Global 1.vi" "술잔 위로 가는 자세"() -> (w378:string)
                n282 = invoke class="PrimaryInterfaceScript" method="Send"(reference=w376, "script"=w378) -> (reference out=w375:refnum<k24>)  [unwired: 2 in, 3 out]
                n283 = Wait (ms)(milliseconds to wait=u32 5000) -> ()  [unwired: 1 out]
              }
              frame #33 {
                # "미니콜라에 따르기"
                n284 = global read "Global 1.vi" "미니콜라 따르는 자세"() -> (w382:string)
                n285 = invoke class="PrimaryInterfaceScript" method="Send"(reference=w380, "script"=w382) -> (reference out=w379:refnum<k24>)  [unwired: 2 in, 3 out]
                n286 = Wait (ms)(milliseconds to wait=u32 11000) -> ()  [unwired: 1 out]
              }
              frame #34 {
                # "술따르기 중단"
                n287 = global read "Global 1.vi" "술잔 위로 가는 자세"() -> (w386:string)
                n288 = invoke class="PrimaryInterfaceScript" method="Send"(reference=w384, "script"=w386) -> (reference out=w383:refnum<k24>)  [unwired: 2 in, 3 out]
                n289 = Wait (ms)(milliseconds to wait=u32 5000) -> ()  [unwired: 1 out]
              }
              frame #35 {
                # "술잔 중간지점으로 이동"
                n290 = global read "Global 1.vi" "술잔 중간지점"() -> (w389:string)
                n291 = invoke class="PrimaryInterfaceScript" method="Send"(reference=w388, "script"=w389) -> (reference out=w387:refnum<k24>)  [unwired: 2 in, 3 out]
                n292 = Wait (ms)(milliseconds to wait=u32 7000) -> ()  [unwired: 1 out]
              }
              frame #36 {
                # "콜라 뻇던 자세로 복귀"
                n293 = global read "Global 1.vi" "콜라 빼는 자세"() -> (w393:string)
                n294 = invoke class="PrimaryInterfaceScript" method="Send"(reference=w392, "script"=w393) -> (reference out=w391:refnum<k24>)  [unwired: 2 in, 3 out]
                n295 = Wait (ms)(milliseconds to wait=u32 7000) -> ()  [unwired: 1 out]
              }
              frame #37 {
                # "콜라 내려놓으러 가기"
                n296 = global read "Global 1.vi" "콜라 드는 자세"() -> (w398:string)
                n297 = invoke class="PrimaryInterfaceScript" method="Send"(reference=w396, "script"=w398) -> (reference out=w395:refnum<k24>)  [unwired: 2 in, 3 out]
                n298 = Wait (ms)(milliseconds to wait=u32 10000) -> ()  [unwired: 1 out]
              }
              frame #38 {
                # "콜라 내려놓기"
                n299 = global read "Global 1.vi" "콜라로 가는자세"() -> (w402:string)
                n300 = invoke class="PrimaryInterfaceScript" method="Send"(reference=w400, "script"=w402) -> (reference out=w399:refnum<k24>)  [unwired: 2 in, 3 out]
                n301 = Wait (ms)(milliseconds to wait=u32 5000) -> ()  [unwired: 1 out]
              }
              frame #39 {
                # "그리퍼 열기"
                n302 = global write "Global 1.vi" "그리퍼 열림"(TRUE ("그리퍼 열림")) -> ()
                n303 = Wait (ms)(milliseconds to wait=u32 300) -> ()  [unwired: 1 out]
              }
              frame #40 {
                n304 = global write "Global 1.vi" "그리퍼 열림"(FALSE ("그리퍼 열림")) -> ()
                n305 = Wait (ms)(milliseconds to wait=u32 3000) -> ()  [unwired: 1 out]
              }
              frame #41 {
                # "콜라 뻇던 자세로 복귀"
                n306 = global read "Global 1.vi" "콜라 빼는 자세"() -> (w411:string)
                n307 = invoke class="PrimaryInterfaceScript" method="Send"(reference=w410, "script"=w411) -> (reference out=w409:refnum<k24>)  [unwired: 2 in, 3 out]
                n308 = Wait (ms)(milliseconds to wait=u32 5000) -> ()  [unwired: 1 out]
              }
              frame #42 {
                # "초기자세"
                n309 = global read "Global 1.vi" "1자로 서는 자세"() -> (w415:string)
                n310 = invoke class="PrimaryInterfaceScript" method="Send"(reference=w413, "script"=w415) -> ()  [unwired: 2 in, 4 out]
                n311 = Wait (ms)(milliseconds to wait=u32 15000) -> ()  [unwired: 1 out]
              }
              frame #43 {
                n312 = global write "Global 1.vi" "그리퍼 닫힘"(TRUE ("그리퍼 열림")) -> ()
                n313 = Wait (ms)(milliseconds to wait=u32 300) -> ()  [unwired: 1 out]
              }
              frame #44 {
                w418 = ""
                # "그리퍼의 앙다문 일자 입"
                n314 = global write "Global 1.vi" "그리퍼 닫힘"(FALSE ("그리퍼 열림")) -> ()
                n315 = Wait (ms)(milliseconds to wait=u32 3000) -> ()  [unwired: 1 out]
                n316 = global write "Global 1.vi" "잭다니엘 카메라 값"(w418) -> ()
                n317 = global write "Global 1.vi" "콜라 카메라 값"(w418) -> ()
                n318 = global write "Global 1.vi" "토닉 카메라 값"(w418) -> ()
                n319 = global write "Global 1.vi" "짐빔 카메라 값"(w418) -> ()
              }
            }
          }
          frame 2 {
            # "짐빔 : 토닉 = 1: 3"
            # "2nd order"
            n320 = flat-sequence {
              tunnel: w433 -> [w464]
              tunnel: [w463] -> w460
              tunnel: w460 -> [w468]
              tunnel: [w466] -> w459
              tunnel: w459 -> [w471]
              tunnel: [w471] -> w458
              tunnel: w458 -> [w474]
              tunnel: [w474] -> w430
              tunnel: w430 -> [w478]
              tunnel: [w478] -> w429
              tunnel: w429 -> [w485]
              tunnel: [w485] -> w428
              tunnel: w428 -> [w561]
              tunnel: [w561] -> w427
              tunnel: w427 -> [w564]
              tunnel: [w564] -> w426
              tunnel: w426 -> [w568]
              tunnel: [w565] -> w457
              tunnel: w457 -> [w571]
              tunnel: [w571] -> w456
              tunnel: w456 -> [w574]
              tunnel: [w574] -> w455
              tunnel: w455 -> [w576]
              tunnel: [w575] -> w454
              tunnel: w454 -> [w580]
              tunnel: [w579] -> w453
              tunnel: w453 -> [w585]
              tunnel: [w583] -> w452
              tunnel: w452 -> [w588]
              tunnel: [w587] -> w451
              tunnel: w451 -> [w593]
              tunnel: [w591] -> w450
              tunnel: w450 -> [w596]
              tunnel: [w595] -> w449
              tunnel: w449 -> [w601]
              tunnel: [w601] -> w448
              tunnel: w448 -> [w604]
              tunnel: [w604] -> w432
              tunnel: w432 -> [w606]
              tunnel: [w605] -> w431
              tunnel: [w609] -> w425
              tunnel: w431 -> [w610]
              tunnel: w425 -> [w616]
              tunnel: [w616] -> w424
              tunnel: w424 -> [w623]
              tunnel: [w623] -> w423
              tunnel: w423 -> [w699]
              tunnel: [w699] -> w422
              tunnel: w422 -> [w702]
              tunnel: [w702] -> w421
              tunnel: w421 -> [w704]
              tunnel: [w703] -> w447
              tunnel: w447 -> [w709]
              tunnel: [w709] -> w446
              tunnel: w446 -> [w712]
              tunnel: [w712] -> w445
              tunnel: w445 -> [w714]
              tunnel: [w713] -> w444
              tunnel: w444 -> [w718]
              tunnel: [w717] -> w443
              tunnel: w443 -> [w722]
              tunnel: [w721] -> w442
              tunnel: w442 -> [w726]
              tunnel: [w725] -> w441
              tunnel: w441 -> [w730]
              tunnel: [w729] -> w440
              tunnel: w440 -> [w734]
              tunnel: [w733] -> w439
              tunnel: w439 -> [w738]
              tunnel: [w737] -> w438
              tunnel: w438 -> [w742]
              tunnel: [w741] -> w437
              tunnel: [w745] -> w436
              tunnel: w437 -> [w745]
              tunnel: [w748] -> w435
              tunnel: w436 -> [w748]
              tunnel: w435 -> [w752]
              tunnel: [w751] -> w434
              tunnel: w434 -> [w755]
              frame #0 {
                # "초기자세"
                n321 = global read "Global 1.vi" "1자로 서는 자세"() -> (w462:string)
                n322 = invoke class="PrimaryInterfaceScript" method="Send"(reference=w464, "script"=w462) -> (reference out=w463:refnum<k24>)  [unwired: 2 in, 3 out]
                n323 = Wait (ms)(milliseconds to wait=u32 15000) -> ()  [unwired: 1 out]
              }
              frame #1 {
                # "짐빔 보기"
                n324 = global read "Global 1.vi" "짐빔 보는 자세"() -> (w467:string)
                n325 = invoke class="PrimaryInterfaceScript" method="Send"(reference=w468, "script"=w467) -> (reference out=w466:refnum<k24>)  [unwired: 2 in, 3 out]
                n326 = Wait (ms)(milliseconds to wait=u32 15000) -> ()  [unwired: 1 out]
              }
              frame #2 {
                # "그리퍼 열기"
                n327 = global write "Global 1.vi" "그리퍼 열림"(TRUE ("그리퍼 열림")) -> ()
                n328 = Wait (ms)(milliseconds to wait=u32 300) -> ()  [unwired: 1 out]
              }
              frame #3 {
                n329 = global write "Global 1.vi" "그리퍼 열림"(FALSE ("그리퍼 열림")) -> ()
                n330 = Wait (ms)(milliseconds to wait=u32 300) -> ()  [unwired: 1 out]
              }
              frame #4 {
                # "tcp 키는 스위치 보단\n파이썬한테 \n값 보내달라하는\n요청 보내는 걸로 \n바꾸기"
                n331 = global write "Global 1.vi" "몇번 병을 볼것인가"("3" ("몇번 병을 볼것인가")) -> ()
                n332 = global write "Global 1.vi" "TCP 스위치"(TRUE ("그리퍼 열림")) -> ()
                n333 = Wait Until Next ms Multiple(millisecond multiple=u32 500 ("milliseconds to wait")) -> ()  [unwired: 1 out]
              }
              frame #5 {
                n334 = global read "Global 1.vi" "X_부호"() -> (w481:string)
                n335 = global read "Global 1.vi" "Z_부호"() -> (w479:string)
                n336 = global read "Global 1.vi" "Y_부호"() -> (w480:string)
                n337 = case shown="\"1\"" w479 {
                  frame "False", Default {
                  }
                  frame "True" {
                  }
                  frame "2" {
                  }
                  frame "1" {
                    n338 = global read "Global 1.vi" "Z_havetogo"() -> (w487:string)
                    n339 = Decimal String To Number(string=w487) -> (number=w490:i32)  [unwired: 2 in, 1 out]
                    n340 = To Double Precision Float(number=w490) -> (double precision float=w489:dbl)
                    n341 = Format Into String(format string="-%f", w489) -> (resulting string=w486:string)  [unwired: 2 in, 1 out]
                    n342 = global write "Global 1.vi" "Z_havetogo"(w486) -> ()
                  }
                }
                n343 = case shown="\"1\"" w480 {
                  frame "False", Default {
                  }
                  frame "True" {
                  }
                  frame "2" {
                  }
                  frame "1" {
                    n344 = global read "Global 1.vi" "Y_havetogo"() -> (w492:string)
                    n345 = Decimal String To Number(string=w492) -> (number=w495:i32)  [unwired: 2 in, 1 out]
                    n346 = To Double Precision Float(number=w495) -> (double precision float=w493:dbl)
                    n347 = Format Into String(format string="-%f", w493) -> (resulting string=w491:string)  [unwired: 2 in, 1 out]
                    n348 = global write "Global 1.vi" "Y_havetogo"(w491) -> ()
                  }
                }
                n349 = case shown="\"1\"" w481 {
                  frame "False", Default {
                  }
                  frame "True" {
                  }
                  frame "2" {
                  }
                  frame "1" {
                    n350 = global read "Global 1.vi" "X_havetogo"() -> (w497:string)
                    n351 = Decimal String To Number(string=w497) -> (number=w500:i32)  [unwired: 2 in, 1 out]
                    n352 = To Double Precision Float(number=w500) -> (double precision float=w499:dbl)
                    n353 = Format Into String(format string="-%f", w499) -> (resulting string=w496:string)  [unwired: 2 in, 1 out]
                    n354 = global write "Global 1.vi" "X_havetogo"(w496) -> ()
                  }
                }
                n355 = global read "Global 1.vi" "RX_부호"() -> (w484:string)
                n356 = global read "Global 1.vi" "RZ_부호"() -> (w482:string)
                n357 = global read "Global 1.vi" "RY_부호"() -> (w483:string)
                n358 = case shown="\"1\"" w482 {
                  frame "False", Default {
                  }
                  frame "True" {
                  }
                  frame "2" {
                  }
                  frame "1" {
                    n359 = global read "Global 1.vi" "RZ_havetogo"() -> (w502:string)
                    n360 = Decimal String To Number(string=w502) -> (number=w505:i32)  [unwired: 2 in, 1 out]
                    n361 = To Double Precision Float(number=w505) -> (double precision float=w504:dbl)
                    n362 = Format Into String(format string="-%f", w504) -> (resulting string=w501:string)  [unwired: 2 in, 1 out]
                    n363 = global write "Global 1.vi" "RZ_havetogo"(w501) -> ()
                  }
                }
                n364 = case shown="\"1\"" w483 {
                  frame "False", Default {
                  }
                  frame "True" {
                  }
                  frame "2" {
                  }
                  frame "1" {
                    n365 = global read "Global 1.vi" "RY_havetogo"() -> (w507:string)
                    n366 = Decimal String To Number(string=w507) -> (number=w510:i32)  [unwired: 2 in, 1 out]
                    n367 = To Double Precision Float(number=w510) -> (double precision float=w508:dbl)
                    n368 = Format Into String(format string="-%f", w508) -> (resulting string=w506:string)  [unwired: 2 in, 1 out]
                    n369 = global write "Global 1.vi" "RY_havetogo"(w506) -> ()
                  }
                }
                n370 = case shown="\"1\"" w484 {
                  frame "False", Default {
                  }
                  frame "True" {
                  }
                  frame "2" {
                  }
                  frame "1" {
                    n371 = global read "Global 1.vi" "RX_havetogo"() -> (w512:string)
                    n372 = Decimal String To Number(string=w512) -> (number=w515:i32)  [unwired: 2 in, 1 out]
                    n373 = To Double Precision Float(number=w515) -> (double precision float=w514:dbl)
                    n374 = Format Into String(format string="-%f", w514) -> (resulting string=w511:string)  [unwired: 2 in, 1 out]
                    n375 = global write "Global 1.vi" "RX_havetogo"(w511) -> ()
                  }
                }
              }
              frame #6 {
                n376 = global read "Global 1.vi" "X_havetogo"() -> (w527:string)
                n377 = global read "Global 1.vi" "Y_havetogo"() -> (w526:string)
                n378 = global read "Global 1.vi" "Z_havetogo"() -> (w525:string)
                n379 = global read "Global 1.vi" "RX_havetogo"() -> (w524:string)
                n380 = global read "Global 1.vi" "RY_havetogo"() -> (w523:string)
                n381 = global read "Global 1.vi" "RZ_havetogo"() -> (w522:string)
                n382 = Decimal String To Number(string=w525) -> (number=w551:i32)  [unwired: 2 in, 1 out]
                n383 = Decimal String To Number(string=w527) -> (number=w557:i32)  [unwired: 2 in, 1 out]
                n384 = Decimal String To Number(string=w526) -> (number=w554:i32)  [unwired: 2 in, 1 out]
                n385 = Decimal String To Number(string=w524) -> (number=w548:i32)  [unwired: 2 in, 1 out]
                n386 = Decimal String To Number(string=w523) -> (number=w545:i32)  [unwired: 2 in, 1 out]
                n387 = Decimal String To Number(string=w522) -> (number=w542:i32)  [unwired: 2 in, 1 out]
                n388 = To Double Precision Float(number=w551) -> (double precision float=w553:dbl)
                n389 = To Double Precision Float(number=w557) -> (double precision float=w559:dbl)
                n390 = To Double Precision Float(number=w554) -> (double precision float=w556:dbl)
                n391 = To Double Precision Float(number=w548) -> (double precision float=w550:dbl)
                n392 = To Double Precision Float(number=w545) -> (double precision float=w547:dbl)
                n393 = Multiply(x=w559, y=0.001) -> (x*y=w541:dbl)
                n394 = Multiply(x=w553, y=0.001) -> (x*y=w537:dbl)
                n395 = Multiply(x=w556, y=0.001) -> (x*y=w539:dbl)
                n396 = Multiply(x=w550, y=0.001) -> (x*y=w535:dbl)
                n397 = global read "Global 1.vi" "x"() -> (w521:dbl)
                n398 = Multiply(x=w547, y=0.001) -> (x*y=w533:dbl)
                n399 = global read "Global 1.vi" "y"() -> (w520:dbl)
                n400 = global read "Global 1.vi" "rx"() -> (w518:dbl)
                n401 = global read "Global 1.vi" "z"() -> (w519:dbl)
                n402 = To Double Precision Float(number=w542) -> (double precision float=w544:dbl)
                n403 = Add(x=w521, y=w541) -> (x+y=w540:dbl)
                n404 = Multiply(x=w544, y=0.001) -> (x*y=w531:dbl)
                n405 = Add(x=w537, y=w519) -> (x+y=w536:dbl)
                n406 = Add(x=w539, y=w520) -> (x+y=w538:dbl)
                n407 = global read "Global 1.vi" "ry"() -> (w516:dbl)
                n408 = global read "Global 1.vi" "rz"() -> (w517:dbl)
                n409 = Add(x=w535, y=w518) -> (x+y=w534:dbl)
                n410 = Add(x=w533, y=w516) -> (x+y=w532:dbl)
                n411 = Add(x=w531, y=w517) -> (x+y=w530:dbl)
                n412 = Format Into String(format string="movej( get_inverse_kin(p[%f, %f, %f, %f, %f, %f]), a= 0.5, v=0.25, t=0, r=0)", w540, w538, w536, w534, w532, w530) -> (resulting string=w528:string)  [unwired: 2 in, 1 out]
                n413 = global write "Global 1.vi" "짐빔 카메라 값"(w528) -> ()
                n414 = Wait (ms)(milliseconds to wait=u32 300) -> ()  [unwired: 1 out]
              }
              frame #7 {
                n415 = global write "Global 1.vi" "TCP 스위치"(FALSE ("그리퍼 열림")) -> ()
                n416 = Wait Until Next ms Multiple(millisecond multiple=u32 300 ("milliseconds to wait")) -> ()  [unwired: 1 out]
              }
              frame #8 {
                # "짐빔 위치로 가기"
                n417 = global read "Global 1.vi" "짐빔 카메라 값"() -> (w567:string)
                n418 = invoke class="PrimaryInterfaceScript" method="Send"(reference=w568, "script"=w567) -> (reference out=w565:refnum<k24>)  [unwired: 2 in, 3 out]
                n419 = Wait (ms)(milliseconds to wait=u32 7000) -> ()  [unwired: 1 out]
              }
              frame #9 {
                # "그리퍼 닫기"
                n420 = global write "Global 1.vi" "그리퍼 닫힘"(TRUE ("그리퍼 열림")) -> ()
                n421 = Wait (ms)(milliseconds to wait=u32 300) -> ()  [unwired: 1 out]
              }
              frame #10 {
                n422 = global write "Global 1.vi" "그리퍼 닫힘"(FALSE ("그리퍼 열림")) -> ()
                n423 = Wait (ms)(milliseconds to wait=u32 3000) -> ()  [unwired: 1 out]
              }
              frame #11 {
                # "짐빔 들기"
                n424 = global read "Global 1.vi" "짐빔 들어올리는 자세"() -> (w578:string)
                n425 = invoke class="PrimaryInterfaceScript" method="Send"(reference=w576, "script"=w578) -> (reference out=w575:refnum<k24>)  [unwired: 2 in, 3 out]
                n426 = Wait (ms)(milliseconds to wait=u32 5000) -> ()  [unwired: 1 out]
              }
              frame #12 {
                # "술잔 쪽으로 이동"
                n427 = global read "Global 1.vi" "술잔 위로 가는 자세 2"() -> (w581:string)
                n428 = invoke class="PrimaryInterfaceScript" method="Send"(reference=w580, "script"=w581) -> (reference out=w579:refnum<k24>)  [unwired: 2 in, 3 out]
                n429 = Wait (ms)(milliseconds to wait=u32 15000) -> ()  [unwired: 1 out]
              }
              frame #13 {
                # "술따르기"
                n430 = global read "Global 1.vi" "술 따르는 자세 2"() -> (w584:string)
                n431 = invoke class="PrimaryInterfaceScript" method="Send"(reference=w585, "script"=w584) -> (reference out=w583:refnum<k24>)  [unwired: 2 in, 3 out]
                n432 = Wait (ms)(milliseconds to wait=u32 9000) -> ()  [unwired: 1 out]
              }
              frame #14 {
                # "술따르기 중단"
                n433 = global read "Global 1.vi" "술잔 위로 가는 자세 2"() -> (w589:string)
                n434 = invoke class="PrimaryInterfaceScript" method="Send"(reference=w588, "script"=w589) -> (reference out=w587:refnum<k24>)  [unwired: 2 in, 3 out]
                n435 = Wait (ms)(milliseconds to wait=u32 4000) -> ()  [unwired: 1 out]
              }
              frame #15 {
                # "짐빔 들었던 곳으로"
                n436 = global read "Global 1.vi" "짐빔 들어올리는 자세"() -> (w592:string)
                n437 = invoke class="PrimaryInterfaceScript" method="Send"(reference=w593, "script"=w592) -> (reference out=w591:refnum<k24>)  [unwired: 2 in, 3 out]
                n438 = Wait (ms)(milliseconds to wait=u32 10000) -> ()  [unwired: 1 out]
              }
              frame #16 {
                # "짐빔 내려놓기"
                n439 = global read "Global 1.vi" "짐빔 위치로 가는 자세"() -> (w598:string)
                n440 = invoke class="PrimaryInterfaceScript" method="Send"(reference=w596, "script"=w598) -> (reference out=w595:refnum<k24>)  [unwired: 2 in, 3 out]
                n441 = Wait (ms)(milliseconds to wait=u32 5000) -> ()  [unwired: 1 out]
              }
              frame #17 {
                # "그리퍼 열기"
                n442 = global write "Global 1.vi" "그리퍼 열림"(TRUE ("그리퍼 열림")) -> ()
                n443 = Wait (ms)(milliseconds to wait=u32 300) -> ()  [unwired: 1 out]
              }
              frame #18 {
                n444 = global write "Global 1.vi" "그리퍼 열림"(FALSE ("그리퍼 열림")) -> ()
                n445 = Wait (ms)(milliseconds to wait=u32 3000) -> ()  [unwired: 1 out]
              }
              frame #19 {
                # "짐빔에서 토닉으로 이동준비"
                n446 = global read "Global 1.vi" "짐빔 토닉 이동 준비자세"() -> (w608:string)
                n447 = invoke class="PrimaryInterfaceScript" method="Send"(reference=w606, "script"=w608) -> (reference out=w605:refnum<k24>)  [unwired: 2 in, 3 out]
                n448 = Wait (ms)(milliseconds to wait=u32 5000) -> ()  [unwired: 1 out]
              }
              frame #20 {
                # "토닉보러가기"
                n449 = global read "Global 1.vi" "토닉 보는 자세"() -> (w612:string)
                n450 = invoke class="PrimaryInterfaceScript" method="Send"(reference=w610, "script"=w612) -> (reference out=w609:refnum<k24>)  [unwired: 2 in, 3 out]
                n451 = Wait (ms)(milliseconds to wait=u32 8000) -> ()  [unwired: 1 out]
              }
              frame #21 {
                # "tcp 키는 스위치 보단\n파이썬한테 \n값 보내달라하는\n요청 보내는 걸로 \n바꾸기"
                n452 = global write "Global 1.vi" "몇번 병을 볼것인가"("4" ("몇번 병을 볼것인가")) -> ()
                n453 = global write "Global 1.vi" "TCP 스위치"(TRUE ("그리퍼 열림")) -> ()
                n454 = Wait Until Next ms Multiple(millisecond multiple=u32 500 ("milliseconds to wait")) -> ()  [unwired: 1 out]
              }
              frame #22 {
                n455 = global read "Global 1.vi" "X_부호"() -> (w619:string)
                n456 = global read "Global 1.vi" "Z_부호"() -> (w617:string)
                n457 = global read "Global 1.vi" "Y_부호"() -> (w618:string)
                n458 = case shown="\"1\"" w617 {
                  frame "False", Default {
                  }
                  frame "True" {
                  }
                  frame "2" {
                  }
                  frame "1" {
                    n459 = global read "Global 1.vi" "Z_havetogo"() -> (w625:string)
                    n460 = Decimal String To Number(string=w625) -> (number=w628:i32)  [unwired: 2 in, 1 out]
                    n461 = To Double Precision Float(number=w628) -> (double precision float=w627:dbl)
                    n462 = Format Into String(format string="-%f", w627) -> (resulting string=w624:string)  [unwired: 2 in, 1 out]
                    n463 = global write "Global 1.vi" "Z_havetogo"(w624) -> ()
                  }
                }
                n464 = case shown="\"1\"" w618 {
                  frame "False", Default {
                  }
                  frame "True" {
                  }
                  frame "2" {
                  }
                  frame "1" {
                    n465 = global read "Global 1.vi" "Y_havetogo"() -> (w630:string)
                    n466 = Decimal String To Number(string=w630) -> (number=w633:i32)  [unwired: 2 in, 1 out]
                    n467 = To Double Precision Float(number=w633) -> (double precision float=w631:dbl)
                    n468 = Format Into String(format string="-%f", w631) -> (resulting string=w629:string)  [unwired: 2 in, 1 out]
                    n469 = global write "Global 1.vi" "Y_havetogo"(w629) -> ()
                  }
                }
                n470 = case shown="\"1\"" w619 {
                  frame "False", Default {
                  }
                  frame "True" {
                  }
                  frame "2" {
                  }
                  frame "1" {
                    n471 = global read "Global 1.vi" "X_havetogo"() -> (w635:string)
                    n472 = Decimal String To Number(string=w635) -> (number=w638:i32)  [unwired: 2 in, 1 out]
                    n473 = To Double Precision Float(number=w638) -> (double precision float=w637:dbl)
                    n474 = Format Into String(format string="-%f", w637) -> (resulting string=w634:string)  [unwired: 2 in, 1 out]
                    n475 = global write "Global 1.vi" "X_havetogo"(w634) -> ()
                  }
                }
                n476 = global read "Global 1.vi" "RX_부호"() -> (w622:string)
                n477 = global read "Global 1.vi" "RZ_부호"() -> (w620:string)
                n478 = global read "Global 1.vi" "RY_부호"() -> (w621:string)
                n479 = case shown="\"1\"" w620 {
                  frame "False", Default {
                  }
                  frame "True" {
                  }
                  frame "2" {
                  }
                  frame "1" {
                    n480 = global read "Global 1.vi" "RZ_havetogo"() -> (w640:string)
                    n481 = Decimal String To Number(string=w640) -> (number=w643:i32)  [unwired: 2 in, 1 out]
                    n482 = To Double Precision Float(number=w643) -> (double precision float=w642:dbl)
                    n483 = Format Into String(format string="-%f", w642) -> (resulting string=w639:string)  [unwired: 2 in, 1 out]
                    n484 = global write "Global 1.vi" "RZ_havetogo"(w639) -> ()
                  }
                }
                n485 = case shown="\"1\"" w621 {
                  frame "False", Default {
                  }
                  frame "True" {
                  }
                  frame "2" {
                  }
                  frame "1" {
                    n486 = global read "Global 1.vi" "RY_havetogo"() -> (w645:string)
                    n487 = Decimal String To Number(string=w645) -> (number=w648:i32)  [unwired: 2 in, 1 out]
                    n488 = To Double Precision Float(number=w648) -> (double precision float=w646:dbl)
                    n489 = Format Into String(format string="-%f", w646) -> (resulting string=w644:string)  [unwired: 2 in, 1 out]
                    n490 = global write "Global 1.vi" "RY_havetogo"(w644) -> ()
                  }
                }
                n491 = case shown="\"1\"" w622 {
                  frame "False", Default {
                  }
                  frame "True" {
                  }
                  frame "2" {
                  }
                  frame "1" {
                    n492 = global read "Global 1.vi" "RX_havetogo"() -> (w650:string)
                    n493 = Decimal String To Number(string=w650) -> (number=w653:i32)  [unwired: 2 in, 1 out]
                    n494 = To Double Precision Float(number=w653) -> (double precision float=w652:dbl)
                    n495 = Format Into String(format string="-%f", w652) -> (resulting string=w649:string)  [unwired: 2 in, 1 out]
                    n496 = global write "Global 1.vi" "RX_havetogo"(w649) -> ()
                  }
                }
              }
              frame #23 {
                n497 = global read "Global 1.vi" "X_havetogo"() -> (w665:string)
                n498 = global read "Global 1.vi" "Y_havetogo"() -> (w664:string)
                n499 = global read "Global 1.vi" "Z_havetogo"() -> (w663:string)
                n500 = global read "Global 1.vi" "RX_havetogo"() -> (w662:string)
                n501 = global read "Global 1.vi" "RY_havetogo"() -> (w661:string)
                n502 = global read "Global 1.vi" "RZ_havetogo"() -> (w660:string)
                n503 = Decimal String To Number(string=w663) -> (number=w689:i32)  [unwired: 2 in, 1 out]
                n504 = Decimal String To Number(string=w665) -> (number=w695:i32)  [unwired: 2 in, 1 out]
                n505 = Decimal String To Number(string=w664) -> (number=w692:i32)  [unwired: 2 in, 1 out]
                n506 = Decimal String To Number(string=w662) -> (number=w686:i32)  [unwired: 2 in, 1 out]
                n507 = Decimal String To Number(string=w661) -> (number=w683:i32)  [unwired: 2 in, 1 out]
                n508 = Decimal String To Number(string=w660) -> (number=w680:i32)  [unwired: 2 in, 1 out]
                n509 = To Double Precision Float(number=w689) -> (double precision float=w691:dbl)
                n510 = To Double Precision Float(number=w695) -> (double precision float=w697:dbl)
                n511 = To Double Precision Float(number=w692) -> (double precision float=w694:dbl)
                n512 = To Double Precision Float(number=w686) -> (double precision float=w688:dbl)
                n513 = To Double Precision Float(number=w683) -> (double precision float=w685:dbl)
                n514 = Multiply(x=w697, y=0.001) -> (x*y=w679:dbl)
                n515 = Multiply(x=w691, y=0.001) -> (x*y=w675:dbl)
                n516 = Multiply(x=w694, y=0.001) -> (x*y=w677:dbl)
                n517 = Multiply(x=w688, y=0.001) -> (x*y=w673:dbl)
                n518 = global read "Global 1.vi" "x"() -> (w659:dbl)
                n519 = Multiply(x=w685, y=0.001) -> (x*y=w671:dbl)
                n520 = global read "Global 1.vi" "y"() -> (w658:dbl)
                n521 = global read "Global 1.vi" "rx"() -> (w656:dbl)
                n522 = global read "Global 1.vi" "z"() -> (w657:dbl)
                n523 = To Double Precision Float(number=w680) -> (double precision float=w682:dbl)
                n524 = Add(x=w659, y=w679) -> (x+y=w678:dbl)
                n525 = Multiply(x=w682, y=0.001) -> (x*y=w669:dbl)
                n526 = Add(x=w675, y=w657) -> (x+y=w674:dbl)
                n527 = Add(x=w677, y=w658) -> (x+y=w676:dbl)
                n528 = global read "Global 1.vi" "ry"() -> (w654:dbl)
                n529 = global read "Global 1.vi" "rz"() -> (w655:dbl)
                n530 = Add(x=w673, y=w656) -> (x+y=w672:dbl)
                n531 = Add(x=w671, y=w654) -> (x+y=w670:dbl)
                n532 = Add(x=w669, y=w655) -> (x+y=w668:dbl)
                n533 = Format Into String(format string="movej( get_inverse_kin(p[%f, %f, %f, %f, %f, %f]), a= 0.5, v=0.25, t=0, r=0)", w678, w676, w674, w672, w670, w668) -> (resulting string=w666:string)  [unwired: 2 in, 1 out]
                n534 = global write "Global 1.vi" "토닉 카메라 값"(w666) -> ()
                n535 = Wait (ms)(milliseconds to wait=u32 300) -> ()  [unwired: 1 out]
              }
              frame #24 {
                n536 = global write "Global 1.vi" "TCP 스위치"(FALSE ("그리퍼 열림")) -> ()
                n537 = Wait Until Next ms Multiple(millisecond multiple=u32 300 ("milliseconds to wait")) -> ()  [unwired: 1 out]
              }
              frame #25 {
                # "토닉 들러가기"
                n538 = global read "Global 1.vi" "토닉 카메라 값"() -> (w706:string)
                n539 = invoke class="PrimaryInterfaceScript" method="Send"(reference=w704, "script"=w706) -> (reference out=w703:refnum<k24>)  [unwired: 2 in, 3 out]
                n540 = Wait (ms)(milliseconds to wait=u32 8000) -> ()  [unwired: 1 out]
              }
              frame #26 {
                n541 = global write "Global 1.vi" "그리퍼 닫힘"(TRUE ("그리퍼 열림")) -> ()
                n542 = Wait (ms)(milliseconds to wait=u32 300) -> ()  [unwired: 1 out]
              }
              frame #27 {
                n543 = global write "Global 1.vi" "그리퍼 닫힘"(FALSE ("그리퍼 열림")) -> ()
                n544 = Wait (ms)(milliseconds to wait=u32 3000) -> ()  [unwired: 1 out]
              }
              frame #28 {
                # "토닉 들어올리기"
                n545 = global read "Global 1.vi" "토닉 드는 자세"() -> (w716:string)
                n546 = invoke class="PrimaryInterfaceScript" method="Send"(reference=w714, "script"=w716) -> (reference out=w713:refnum<k24>)  [unwired: 2 in, 3 out]
                n547 = Wait (ms)(milliseconds to wait=u32 5000) -> ()  [unwired: 1 out]
              }
              frame #29 {
                # "토닉 살짝 빼기"
                n548 = global read "Global 1.vi" "토닉 빼는 자세"() -> (w720:string)
                n549 = invoke class="PrimaryInterfaceScript" method="Send"(reference=w718, "script"=w720) -> (reference out=w717:refnum<k24>)  [unwired: 2 in, 3 out]
                n550 = Wait (ms)(milliseconds to wait=u32 7000) -> ()  [unwired: 1 out]
              }
              frame #30 {
                # "술잔으로 이동"
                n551 = global read "Global 1.vi" "술잔 위로 가는 자세 2"() -> (w724:string)
                n552 = invoke class="PrimaryInterfaceScript" method="Send"(reference=w722, "script"=w724) -> (reference out=w721:refnum<k24>)  [unwired: 2 in, 3 out]
                n553 = Wait (ms)(milliseconds to wait=u32 12000) -> ()  [unwired: 1 out]
              }
              frame #31 {
                # "술잔에 따르기"
                n554 = global read "Global 1.vi" "술 따르는 자세 2"() -> (w728:string)
                n555 = invoke class="PrimaryInterfaceScript" method="Send"(reference=w726, "script"=w728) -> (reference out=w725:refnum<k24>)  [unwired: 2 in, 3 out]
                n556 = Wait (ms)(milliseconds to wait=u32 13000) -> ()  [unwired: 1 out]
              }
              frame #32 {
                # "술따르기 중단"
                n557 = global read "Global 1.vi" "술잔 위로 가는 자세 2"() -> (w732:string)
                n558 = invoke class="PrimaryInterfaceScript" method="Send"(reference=w730, "script"=w732) -> (reference out=w729:refnum<k24>)  [unwired: 2 in, 3 out]
                n559 = Wait (ms)(milliseconds to wait=u32 5000) -> ()  [unwired: 1 out]
              }
              frame #33 {
                # "토닉 뻇던 자세로 복귀"
                n560 = global read "Global 1.vi" "토닉 빼는 자세"() -> (w735:string)
                n561 = invoke class="PrimaryInterfaceScript" method="Send"(reference=w734, "script"=w735) -> (reference out=w733:refnum<k24>)  [unwired: 2 in, 3 out]
                n562 = Wait (ms)(milliseconds to wait=u32 9000) -> ()  [unwired: 1 out]
              }
              frame #34 {
                # "토닉 내려놓으러 가기"
                n563 = global read "Global 1.vi" "토닉 드는 자세"() -> (w740:string)
                n564 = invoke class="PrimaryInterfaceScript" method="Send"(reference=w738, "script"=w740) -> (reference out=w737:refnum<k24>)  [unwired: 2 in, 3 out]
                n565 = Wait (ms)(milliseconds to wait=u32 7000) -> ()  [unwired: 1 out]
              }
              frame #35 {
                # "토닉 내려놓기"
                n566 = global read "Global 1.vi" "토닉 가는자세"() -> (w744:string)
                n567 = invoke class="PrimaryInterfaceScript" method="Send"(reference=w742, "script"=w744) -> (reference out=w741:refnum<k24>)  [unwired: 2 in, 3 out]
                n568 = Wait (ms)(milliseconds to wait=u32 5000) -> ()  [unwired: 1 out]
              }
              frame #36 {
                # "그리퍼 열기"
                n569 = global write "Global 1.vi" "그리퍼 열림"(TRUE ("그리퍼 열림")) -> ()
                n570 = Wait (ms)(milliseconds to wait=u32 300) -> ()  [unwired: 1 out]
              }
              frame #37 {
                n571 = global write "Global 1.vi" "그리퍼 열림"(FALSE ("그리퍼 열림")) -> ()
                n572 = Wait (ms)(milliseconds to wait=u32 3000) -> ()  [unwired: 1 out]
              }
              frame #38 {
                # "토닉 뻇던 자세로 복귀"
                n573 = global read "Global 1.vi" "토닉 빼는 자세"() -> (w753:string)
                n574 = invoke class="PrimaryInterfaceScript" method="Send"(reference=w752, "script"=w753) -> (reference out=w751:refnum<k24>)  [unwired: 2 in, 3 out]
                n575 = Wait (ms)(milliseconds to wait=u32 5000) -> ()  [unwired: 1 out]
              }
              frame #39 {
                # "초기자세"
                n576 = global read "Global 1.vi" "1자로 서는 자세"() -> (w757:string)
                n577 = invoke class="PrimaryInterfaceScript" method="Send"(reference=w755, "script"=w757) -> ()  [unwired: 2 in, 4 out]
                n578 = Wait (ms)(milliseconds to wait=u32 15000) -> ()  [unwired: 1 out]
              }
              frame #40 {
                n579 = global write "Global 1.vi" "그리퍼 닫힘"(TRUE ("그리퍼 열림")) -> ()
                n580 = Wait (ms)(milliseconds to wait=u32 300) -> ()  [unwired: 1 out]
              }
              frame #41 {
                w760 = ""
                # "그리퍼의 앙다문 일자 입"
                n581 = global write "Global 1.vi" "그리퍼 닫힘"(FALSE ("그리퍼 열림")) -> ()
                n582 = Wait (ms)(milliseconds to wait=u32 3000) -> ()  [unwired: 1 out]
                n583 = global write "Global 1.vi" "잭다니엘 카메라 값"(w760) -> ()
                n584 = global write "Global 1.vi" "콜라 카메라 값"(w760) -> ()
                n585 = global write "Global 1.vi" "토닉 카메라 값"(w760) -> ()
                n586 = global write "Global 1.vi" "짐빔 카메라 값"(w760) -> ()
              }
            }
          }
          frame 3 {
            # "multi order"
          }
          frame 4 {
            # "짐빔 : 우유 = 1 : 3"
            # "3rd order"
            n587 = flat-sequence {
              tunnel: w763 -> [w806]
              tunnel: [w805] -> w802
              tunnel: w802 -> [w810]
              tunnel: [w808] -> w801
              tunnel: w801 -> [w813]
              tunnel: [w813] -> w800
              tunnel: w800 -> [w816]
              tunnel: [w816] -> w799
              tunnel: w799 -> [w820]
              tunnel: [w820] -> w798
              tunnel: w798 -> [w827]
              tunnel: [w827] -> w797
              tunnel: w797 -> [w903]
              tunnel: [w903] -> w796
              tunnel: w796 -> [w906]
              tunnel: [w906] -> w795
              tunnel: w795 -> [w910]
              tunnel: [w907] -> w794
              tunnel: w794 -> [w913]
              tunnel: [w913] -> w793
              tunnel: w793 -> [w916]
              tunnel: [w916] -> w792
              tunnel: w792 -> [w918]
              tunnel: [w917] -> w791
              tunnel: w791 -> [w922]
              tunnel: [w921] -> w790
              tunnel: w790 -> [w927]
              tunnel: [w925] -> w789
              tunnel: w789 -> [w930]
              tunnel: [w929] -> w788
              tunnel: w788 -> [w935]
              tunnel: [w933] -> w787
              tunnel: w787 -> [w938]
              tunnel: [w937] -> w786
              tunnel: w786 -> [w943]
              tunnel: [w943] -> w785
              tunnel: w785 -> [w946]
              tunnel: [w946] -> w784
              tunnel: w784 -> [w948]
              tunnel: [w947] -> w783
              tunnel: [w951] -> w782
              tunnel: w783 -> [w952]
              tunnel: w782 -> [w958]
              tunnel: [w958] -> w781
              tunnel: w781 -> [w965]
              tunnel: [w965] -> w780
              tunnel: w780 -> [w1041]
              tunnel: [w1041] -> w779
              tunnel: w779 -> [w1044]
              tunnel: [w1044] -> w778
              tunnel: w778 -> [w1046]
              tunnel: [w1045] -> w777
              tunnel: w777 -> [w1051]
              tunnel: [w1051] -> w776
              tunnel: w776 -> [w1054]
              tunnel: [w1054] -> w775
              tunnel: w775 -> [w1056]
              tunnel: [w1055] -> w774
              tunnel: w774 -> [w1060]
              tunnel: [w1059] -> w773
              tunnel: w773 -> [w1064]
              tunnel: [w1063] -> w772
              tunnel: w772 -> [w1068]
              tunnel: [w1067] -> w771
              tunnel: w771 -> [w1072]
              tunnel: [w1071] -> w770
              tunnel: w770 -> [w1076]
              tunnel: [w1075] -> w769
              tunnel: w769 -> [w1080]
              tunnel: [w1079] -> w768
              tunnel: w768 -> [w1084]
              tunnel: [w1083] -> w767
              tunnel: [w1087] -> w766
              tunnel: w767 -> [w1087]
              tunnel: [w1090] -> w765
              tunnel: w766 -> [w1090]
              tunnel: w765 -> [w1094]
              tunnel: [w1093] -> w764
              tunnel: w764 -> [w1097]
              frame #0 {
                # "초기자세"
                n588 = global read "Global 1.vi" "1자로 서는 자세"() -> (w804:string)
                n589 = invoke class="PrimaryInterfaceScript" method="Send"(reference=w806, "script"=w804) -> (reference out=w805:refnum<k24>)  [unwired: 2 in, 3 out]
                n590 = Wait (ms)(milliseconds to wait=u32 15000) -> ()  [unwired: 1 out]
              }
              frame #1 {
                # "짐빔 보기"
                n591 = global read "Global 1.vi" "짐빔 보는 자세"() -> (w809:string)
                n592 = invoke class="PrimaryInterfaceScript" method="Send"(reference=w810, "script"=w809) -> (reference out=w808:refnum<k24>)  [unwired: 2 in, 3 out]
                n593 = Wait (ms)(milliseconds to wait=u32 15000) -> ()  [unwired: 1 out]
              }
              frame #2 {
                # "그리퍼 열기"
                n594 = global write "Global 1.vi" "그리퍼 열림"(TRUE ("그리퍼 열림")) -> ()
                n595 = Wait (ms)(milliseconds to wait=u32 300) -> ()  [unwired: 1 out]
              }
              frame #3 {
                n596 = global write "Global 1.vi" "그리퍼 열림"(FALSE ("그리퍼 열림")) -> ()
                n597 = Wait (ms)(milliseconds to wait=u32 300) -> ()  [unwired: 1 out]
              }
              frame #4 {
                # "tcp 키는 스위치 보단\n파이썬한테 \n값 보내달라하는\n요청 보내는 걸로 \n바꾸기"
                n598 = global write "Global 1.vi" "몇번 병을 볼것인가"("3" ("몇번 병을 볼것인가")) -> ()
                n599 = global write "Global 1.vi" "TCP 스위치"(TRUE ("그리퍼 열림")) -> ()
                n600 = Wait Until Next ms Multiple(millisecond multiple=u32 500 ("milliseconds to wait")) -> ()  [unwired: 1 out]
              }
              frame #5 {
                n601 = global read "Global 1.vi" "X_부호"() -> (w823:string)
                n602 = global read "Global 1.vi" "Z_부호"() -> (w821:string)
                n603 = global read "Global 1.vi" "Y_부호"() -> (w822:string)
                n604 = case shown="\"1\"" w821 {
                  frame "False", Default {
                  }
                  frame "True" {
                  }
                  frame "2" {
                  }
                  frame "1" {
                    n605 = global read "Global 1.vi" "Z_havetogo"() -> (w829:string)
                    n606 = Decimal String To Number(string=w829) -> (number=w832:i32)  [unwired: 2 in, 1 out]
                    n607 = To Double Precision Float(number=w832) -> (double precision float=w831:dbl)
                    n608 = Format Into String(format string="-%f", w831) -> (resulting string=w828:string)  [unwired: 2 in, 1 out]
                    n609 = global write "Global 1.vi" "Z_havetogo"(w828) -> ()
                  }
                }
                n610 = case shown="\"1\"" w822 {
                  frame "False", Default {
                  }
                  frame "True" {
                  }
                  frame "2" {
                  }
                  frame "1" {
                    n611 = global read "Global 1.vi" "Y_havetogo"() -> (w834:string)
                    n612 = Decimal String To Number(string=w834) -> (number=w837:i32)  [unwired: 2 in, 1 out]
                    n613 = To Double Precision Float(number=w837) -> (double precision float=w835:dbl)
                    n614 = Format Into String(format string="-%f", w835) -> (resulting string=w833:string)  [unwired: 2 in, 1 out]
                    n615 = global write "Global 1.vi" "Y_havetogo"(w833) -> ()
                  }
                }
                n616 = case shown="\"1\"" w823 {
                  frame "False", Default {
                  }
                  frame "True" {
                  }
                  frame "2" {
                  }
                  frame "1" {
                    n617 = global read "Global 1.vi" "X_havetogo"() -> (w839:string)
                    n618 = Decimal String To Number(string=w839) -> (number=w842:i32)  [unwired: 2 in, 1 out]
                    n619 = To Double Precision Float(number=w842) -> (double precision float=w841:dbl)
                    n620 = Format Into String(format string="-%f", w841) -> (resulting string=w838:string)  [unwired: 2 in, 1 out]
                    n621 = global write "Global 1.vi" "X_havetogo"(w838) -> ()
                  }
                }
                n622 = global read "Global 1.vi" "RX_부호"() -> (w826:string)
                n623 = global read "Global 1.vi" "RZ_부호"() -> (w824:string)
                n624 = global read "Global 1.vi" "RY_부호"() -> (w825:string)
                n625 = case shown="\"1\"" w824 {
                  frame "False", Default {
                  }
                  frame "True" {
                  }
                  frame "2" {
                  }
                  frame "1" {
                    n626 = global read "Global 1.vi" "RZ_havetogo"() -> (w844:string)
                    n627 = Decimal String To Number(string=w844) -> (number=w847:i32)  [unwired: 2 in, 1 out]
                    n628 = To Double Precision Float(number=w847) -> (double precision float=w846:dbl)
                    n629 = Format Into String(format string="-%f", w846) -> (resulting string=w843:string)  [unwired: 2 in, 1 out]
                    n630 = global write "Global 1.vi" "RZ_havetogo"(w843) -> ()
                  }
                }
                n631 = case shown="\"1\"" w825 {
                  frame "False", Default {
                  }
                  frame "True" {
                  }
                  frame "2" {
                  }
                  frame "1" {
                    n632 = global read "Global 1.vi" "RY_havetogo"() -> (w849:string)
                    n633 = Decimal String To Number(string=w849) -> (number=w852:i32)  [unwired: 2 in, 1 out]
                    n634 = To Double Precision Float(number=w852) -> (double precision float=w850:dbl)
                    n635 = Format Into String(format string="-%f", w850) -> (resulting string=w848:string)  [unwired: 2 in, 1 out]
                    n636 = global write "Global 1.vi" "RY_havetogo"(w848) -> ()
                  }
                }
                n637 = case shown="\"1\"" w826 {
                  frame "False", Default {
                  }
                  frame "True" {
                  }
                  frame "2" {
                  }
                  frame "1" {
                    n638 = global read "Global 1.vi" "RX_havetogo"() -> (w854:string)
                    n639 = Decimal String To Number(string=w854) -> (number=w857:i32)  [unwired: 2 in, 1 out]
                    n640 = To Double Precision Float(number=w857) -> (double precision float=w856:dbl)
                    n641 = Format Into String(format string="-%f", w856) -> (resulting string=w853:string)  [unwired: 2 in, 1 out]
                    n642 = global write "Global 1.vi" "RX_havetogo"(w853) -> ()
                  }
                }
              }
              frame #6 {
                n643 = global read "Global 1.vi" "X_havetogo"() -> (w869:string)
                n644 = global read "Global 1.vi" "Y_havetogo"() -> (w868:string)
                n645 = global read "Global 1.vi" "Z_havetogo"() -> (w867:string)
                n646 = global read "Global 1.vi" "RX_havetogo"() -> (w866:string)
                n647 = global read "Global 1.vi" "RY_havetogo"() -> (w865:string)
                n648 = global read "Global 1.vi" "RZ_havetogo"() -> (w864:string)
                n649 = Decimal String To Number(string=w867) -> (number=w893:i32)  [unwired: 2 in, 1 out]
                n650 = Decimal String To Number(string=w869) -> (number=w899:i32)  [unwired: 2 in, 1 out]
                n651 = Decimal String To Number(string=w868) -> (number=w896:i32)  [unwired: 2 in, 1 out]
                n652 = Decimal String To Number(string=w866) -> (number=w890:i32)  [unwired: 2 in, 1 out]
                n653 = Decimal String To Number(string=w865) -> (number=w887:i32)  [unwired: 2 in, 1 out]
                n654 = Decimal String To Number(string=w864) -> (number=w884:i32)  [unwired: 2 in, 1 out]
                n655 = To Double Precision Float(number=w893) -> (double precision float=w895:dbl)
                n656 = To Double Precision Float(number=w899) -> (double precision float=w901:dbl)
                n657 = To Double Precision Float(number=w896) -> (double precision float=w898:dbl)
                n658 = To Double Precision Float(number=w890) -> (double precision float=w892:dbl)
                n659 = To Double Precision Float(number=w887) -> (double precision float=w889:dbl)
                n660 = Multiply(x=w901, y=0.001) -> (x*y=w883:dbl)
                n661 = Multiply(x=w895, y=0.001) -> (x*y=w879:dbl)
                n662 = Multiply(x=w898, y=0.001) -> (x*y=w881:dbl)
                n663 = Multiply(x=w892, y=0.001) -> (x*y=w877:dbl)
                n664 = global read "Global 1.vi" "x"() -> (w863:dbl)
                n665 = Multiply(x=w889, y=0.001) -> (x*y=w875:dbl)
                n666 = global read "Global 1.vi" "y"() -> (w862:dbl)
                n667 = global read "Global 1.vi" "rx"() -> (w860:dbl)
                n668 = global read "Global 1.vi" "z"() -> (w861:dbl)
                n669 = To Double Precision Float(number=w884) -> (double precision float=w886:dbl)
                n670 = Add(x=w863, y=w883) -> (x+y=w882:dbl)
                n671 = Multiply(x=w886, y=0.001) -> (x*y=w873:dbl)
                n672 = Add(x=w879, y=w861) -> (x+y=w878:dbl)
                n673 = Add(x=w881, y=w862) -> (x+y=w880:dbl)
                n674 = global read "Global 1.vi" "ry"() -> (w858:dbl)
                n675 = global read "Global 1.vi" "rz"() -> (w859:dbl)
                n676 = Add(x=w877, y=w860) -> (x+y=w876:dbl)
                n677 = Add(x=w875, y=w858) -> (x+y=w874:dbl)
                n678 = Add(x=w873, y=w859) -> (x+y=w872:dbl)
                n679 = Format Into String(format string="movej( get_inverse_kin(p[%f, %f, %f, %f, %f, %f]), a= 0.5, v=0.25, t=0, r=0)", w882, w880, w878, w876, w874, w872) -> (resulting string=w870:string)  [unwired: 2 in, 1 out]
                n680 = global write "Global 1.vi" "짐빔 카메라 값"(w870) -> ()
                n681 = Wait (ms)(milliseconds to wait=u32 300) -> ()  [unwired: 1 out]
              }
              frame #7 {
                n682 = global write "Global 1.vi" "TCP 스위치"(FALSE ("그리퍼 열림")) -> ()
                n683 = Wait Until Next ms Multiple(millisecond multiple=u32 300 ("milliseconds to wait")) -> ()  [unwired: 1 out]
              }
              frame #8 {
                # "짐빔 위치로 가기"
                n684 = global read "Global 1.vi" "짐빔 카메라 값"() -> (w909:string)
                n685 = invoke class="PrimaryInterfaceScript" method="Send"(reference=w910, "script"=w909) -> (reference out=w907:refnum<k24>)  [unwired: 2 in, 3 out]
                n686 = Wait (ms)(milliseconds to wait=u32 7000) -> ()  [unwired: 1 out]
              }
              frame #9 {
                # "그리퍼 닫기"
                n687 = global write "Global 1.vi" "그리퍼 닫힘"(TRUE ("그리퍼 열림")) -> ()
                n688 = Wait (ms)(milliseconds to wait=u32 300) -> ()  [unwired: 1 out]
              }
              frame #10 {
                n689 = global write "Global 1.vi" "그리퍼 닫힘"(FALSE ("그리퍼 열림")) -> ()
                n690 = Wait (ms)(milliseconds to wait=u32 3000) -> ()  [unwired: 1 out]
              }
              frame #11 {
                # "짐빔 들기"
                n691 = global read "Global 1.vi" "짐빔 들어올리는 자세"() -> (w920:string)
                n692 = invoke class="PrimaryInterfaceScript" method="Send"(reference=w918, "script"=w920) -> (reference out=w917:refnum<k24>)  [unwired: 2 in, 3 out]
                n693 = Wait (ms)(milliseconds to wait=u32 5000) -> ()  [unwired: 1 out]
              }
              frame #12 {
                # "술잔 쪽으로 이동"
                n694 = global read "Global 1.vi" "술잔 위로 가는 자세 2"() -> (w923:string)
                n695 = invoke class="PrimaryInterfaceScript" method="Send"(reference=w922, "script"=w923) -> (reference out=w921:refnum<k24>)  [unwired: 2 in, 3 out]
                n696 = Wait (ms)(milliseconds to wait=u32 15000) -> ()  [unwired: 1 out]
              }
              frame #13 {
                # "술따르기"
                n697 = global read "Global 1.vi" "술 따르는 자세 2"() -> (w926:string)
                n698 = invoke class="PrimaryInterfaceScript" method="Send"(reference=w927, "script"=w926) -> (reference out=w925:refnum<k24>)  [unwired: 2 in, 3 out]
                n699 = Wait (ms)(milliseconds to wait=u32 9000) -> ()  [unwired: 1 out]
              }
              frame #14 {
                # "술따르기 중단"
                n700 = global read "Global 1.vi" "술잔 위로 가는 자세 2"() -> (w931:string)
                n701 = invoke class="PrimaryInterfaceScript" method="Send"(reference=w930, "script"=w931) -> (reference out=w929:refnum<k24>)  [unwired: 2 in, 3 out]
                n702 = Wait (ms)(milliseconds to wait=u32 4000) -> ()  [unwired: 1 out]
              }
              frame #15 {
                # "짐빔 들었던 곳으로"
                n703 = global read "Global 1.vi" "짐빔 들어올리는 자세"() -> (w934:string)
                n704 = invoke class="PrimaryInterfaceScript" method="Send"(reference=w935, "script"=w934) -> (reference out=w933:refnum<k24>)  [unwired: 2 in, 3 out]
                n705 = Wait (ms)(milliseconds to wait=u32 10000) -> ()  [unwired: 1 out]
              }
              frame #16 {
                # "짐빔 내려놓기"
                n706 = global read "Global 1.vi" "짐빔 위치로 가는 자세"() -> (w940:string)
                n707 = invoke class="PrimaryInterfaceScript" method="Send"(reference=w938, "script"=w940) -> (reference out=w937:refnum<k24>)  [unwired: 2 in, 3 out]
                n708 = Wait (ms)(milliseconds to wait=u32 5000) -> ()  [unwired: 1 out]
              }
              frame #17 {
                # "그리퍼 열기"
                n709 = global write "Global 1.vi" "그리퍼 열림"(TRUE ("그리퍼 열림")) -> ()
                n710 = Wait (ms)(milliseconds to wait=u32 300) -> ()  [unwired: 1 out]
              }
              frame #18 {
                n711 = global write "Global 1.vi" "그리퍼 열림"(FALSE ("그리퍼 열림")) -> ()
                n712 = Wait (ms)(milliseconds to wait=u32 3000) -> ()  [unwired: 1 out]
              }
              frame #19 {
                # "짐빔에서 토닉으로 이동준비"
                n713 = global read "Global 1.vi" "짐빔 토닉 이동 준비자세"() -> (w950:string)
                n714 = invoke class="PrimaryInterfaceScript" method="Send"(reference=w948, "script"=w950) -> (reference out=w947:refnum<k24>)  [unwired: 2 in, 3 out]
                n715 = Wait (ms)(milliseconds to wait=u32 5000) -> ()  [unwired: 1 out]
              }
              frame #20 {
                # "토닉보러가기"
                n716 = global read "Global 1.vi" "토닉 보는 자세"() -> (w954:string)
                n717 = invoke class="PrimaryInterfaceScript" method="Send"(reference=w952, "script"=w954) -> (reference out=w951:refnum<k24>)  [unwired: 2 in, 3 out]
                n718 = Wait (ms)(milliseconds to wait=u32 8000) -> ()  [unwired: 1 out]
              }
              frame #21 {
                # "tcp 키는 스위치 보단\n파이썬한테 \n값 보내달라하는\n요청 보내는 걸로 \n바꾸기"
                n719 = global write "Global 1.vi" "몇번 병을 볼것인가"("4" ("몇번 병을 볼것인가")) -> ()
                n720 = global write "Global 1.vi" "TCP 스위치"(TRUE ("그리퍼 열림")) -> ()
                n721 = Wait Until Next ms Multiple(millisecond multiple=u32 500 ("milliseconds to wait")) -> ()  [unwired: 1 out]
              }
              frame #22 {
                n722 = global read "Global 1.vi" "X_부호"() -> (w961:string)
                n723 = global read "Global 1.vi" "Z_부호"() -> (w959:string)
                n724 = global read "Global 1.vi" "Y_부호"() -> (w960:string)
                n725 = case shown="\"1\"" w959 {
                  frame "False", Default {
                  }
                  frame "True" {
                  }
                  frame "2" {
                  }
                  frame "1" {
                    n726 = global read "Global 1.vi" "Z_havetogo"() -> (w967:string)
                    n727 = Decimal String To Number(string=w967) -> (number=w970:i32)  [unwired: 2 in, 1 out]
                    n728 = To Double Precision Float(number=w970) -> (double precision float=w969:dbl)
                    n729 = Format Into String(format string="-%f", w969) -> (resulting string=w966:string)  [unwired: 2 in, 1 out]
                    n730 = global write "Global 1.vi" "Z_havetogo"(w966) -> ()
                  }
                }
                n731 = case shown="\"1\"" w960 {
                  frame "False", Default {
                  }
                  frame "True" {
                  }
                  frame "2" {
                  }
                  frame "1" {
                    n732 = global read "Global 1.vi" "Y_havetogo"() -> (w972:string)
                    n733 = Decimal String To Number(string=w972) -> (number=w975:i32)  [unwired: 2 in, 1 out]
                    n734 = To Double Precision Float(number=w975) -> (double precision float=w973:dbl)
                    n735 = Format Into String(format string="-%f", w973) -> (resulting string=w971:string)  [unwired: 2 in, 1 out]
                    n736 = global write "Global 1.vi" "Y_havetogo"(w971) -> ()
                  }
                }
                n737 = case shown="\"1\"" w961 {
                  frame "False", Default {
                  }
                  frame "True" {
                  }
                  frame "2" {
                  }
                  frame "1" {
                    n738 = global read "Global 1.vi" "X_havetogo"() -> (w977:string)
                    n739 = Decimal String To Number(string=w977) -> (number=w980:i32)  [unwired: 2 in, 1 out]
                    n740 = To Double Precision Float(number=w980) -> (double precision float=w979:dbl)
                    n741 = Format Into String(format string="-%f", w979) -> (resulting string=w976:string)  [unwired: 2 in, 1 out]
                    n742 = global write "Global 1.vi" "X_havetogo"(w976) -> ()
                  }
                }
                n743 = global read "Global 1.vi" "RX_부호"() -> (w964:string)
                n744 = global read "Global 1.vi" "RZ_부호"() -> (w962:string)
                n745 = global read "Global 1.vi" "RY_부호"() -> (w963:string)
                n746 = case shown="\"1\"" w962 {
                  frame "False", Default {
                  }
                  frame "True" {
                  }
                  frame "2" {
                  }
                  frame "1" {
                    n747 = global read "Global 1.vi" "RZ_havetogo"() -> (w982:string)
                    n748 = Decimal String To Number(string=w982) -> (number=w985:i32)  [unwired: 2 in, 1 out]
                    n749 = To Double Precision Float(number=w985) -> (double precision float=w984:dbl)
                    n750 = Format Into String(format string="-%f", w984) -> (resulting string=w981:string)  [unwired: 2 in, 1 out]
                    n751 = global write "Global 1.vi" "RZ_havetogo"(w981) -> ()
                  }
                }
                n752 = case shown="\"1\"" w963 {
                  frame "False", Default {
                  }
                  frame "True" {
                  }
                  frame "2" {
                  }
                  frame "1" {
                    n753 = global read "Global 1.vi" "RY_havetogo"() -> (w987:string)
                    n754 = Decimal String To Number(string=w987) -> (number=w990:i32)  [unwired: 2 in, 1 out]
                    n755 = To Double Precision Float(number=w990) -> (double precision float=w988:dbl)
                    n756 = Format Into String(format string="-%f", w988) -> (resulting string=w986:string)  [unwired: 2 in, 1 out]
                    n757 = global write "Global 1.vi" "RY_havetogo"(w986) -> ()
                  }
                }
                n758 = case shown="\"1\"" w964 {
                  frame "False", Default {
                  }
                  frame "True" {
                  }
                  frame "2" {
                  }
                  frame "1" {
                    n759 = global read "Global 1.vi" "RX_havetogo"() -> (w992:string)
                    n760 = Decimal String To Number(string=w992) -> (number=w995:i32)  [unwired: 2 in, 1 out]
                    n761 = To Double Precision Float(number=w995) -> (double precision float=w994:dbl)
                    n762 = Format Into String(format string="-%f", w994) -> (resulting string=w991:string)  [unwired: 2 in, 1 out]
                    n763 = global write "Global 1.vi" "RX_havetogo"(w991) -> ()
                  }
                }
              }
              frame #23 {
                n764 = global read "Global 1.vi" "X_havetogo"() -> (w1007:string)
                n765 = global read "Global 1.vi" "Y_havetogo"() -> (w1006:string)
                n766 = global read "Global 1.vi" "Z_havetogo"() -> (w1005:string)
                n767 = global read "Global 1.vi" "RX_havetogo"() -> (w1004:string)
                n768 = global read "Global 1.vi" "RY_havetogo"() -> (w1003:string)
                n769 = global read "Global 1.vi" "RZ_havetogo"() -> (w1002:string)
                n770 = Decimal String To Number(string=w1005) -> (number=w1031:i32)  [unwired: 2 in, 1 out]
                n771 = Decimal String To Number(string=w1007) -> (number=w1037:i32)  [unwired: 2 in, 1 out]
                n772 = Decimal String To Number(string=w1006) -> (number=w1034:i32)  [unwired: 2 in, 1 out]
                n773 = Decimal String To Number(string=w1004) -> (number=w1028:i32)  [unwired: 2 in, 1 out]
                n774 = Decimal String To Number(string=w1003) -> (number=w1025:i32)  [unwired: 2 in, 1 out]
                n775 = Decimal String To Number(string=w1002) -> (number=w1022:i32)  [unwired: 2 in, 1 out]
                n776 = To Double Precision Float(number=w1031) -> (double precision float=w1033:dbl)
                n777 = To Double Precision Float(number=w1037) -> (double precision float=w1039:dbl)
                n778 = To Double Precision Float(number=w1034) -> (double precision float=w1036:dbl)
                n779 = To Double Precision Float(number=w1028) -> (double precision float=w1030:dbl)
                n780 = To Double Precision Float(number=w1025) -> (double precision float=w1027:dbl)
                n781 = Multiply(x=w1039, y=0.001) -> (x*y=w1021:dbl)
                n782 = Multiply(x=w1033, y=0.001) -> (x*y=w1017:dbl)
                n783 = Multiply(x=w1036, y=0.001) -> (x*y=w1019:dbl)
                n784 = Multiply(x=w1030, y=0.001) -> (x*y=w1015:dbl)
                n785 = global read "Global 1.vi" "x"() -> (w1001:dbl)
                n786 = Multiply(x=w1027, y=0.001) -> (x*y=w1013:dbl)
                n787 = global read "Global 1.vi" "y"() -> (w1000:dbl)
                n788 = global read "Global 1.vi" "rx"() -> (w998:dbl)
                n789 = global read "Global 1.vi" "z"() -> (w999:dbl)
                n790 = To Double Precision Float(number=w1022) -> (double precision float=w1024:dbl)
                n791 = Add(x=w1001, y=w1021) -> (x+y=w1020:dbl)
                n792 = Multiply(x=w1024, y=0.001) -> (x*y=w1011:dbl)
                n793 = Add(x=w1017, y=w999) -> (x+y=w1016:dbl)
                n794 = Add(x=w1019, y=w1000) -> (x+y=w1018:dbl)
                n795 = global read "Global 1.vi" "ry"() -> (w996:dbl)
                n796 = global read "Global 1.vi" "rz"() -> (w997:dbl)
                n797 = Add(x=w1015, y=w998) -> (x+y=w1014:dbl)
                n798 = Add(x=w1013, y=w996) -> (x+y=w1012:dbl)
                n799 = Add(x=w1011, y=w997) -> (x+y=w1010:dbl)
                n800 = Format Into String(format string="movej( get_inverse_kin(p[%f, %f, %f, %f, %f, %f]), a= 0.5, v=0.25, t=0, r=0)", w1020, w1018, w1016, w1014, w1012, w1010) -> (resulting string=w1008:string)  [unwired: 2 in, 1 out]
                n801 = global write "Global 1.vi" "토닉 카메라 값"(w1008) -> ()
                n802 = Wait (ms)(milliseconds to wait=u32 300) -> ()  [unwired: 1 out]
              }
              frame #24 {
                n803 = global write "Global 1.vi" "TCP 스위치"(FALSE ("그리퍼 열림")) -> ()
                n804 = Wait Until Next ms Multiple(millisecond multiple=u32 300 ("milliseconds to wait")) -> ()  [unwired: 1 out]
              }
              frame #25 {
                # "토닉 들러가기"
                n805 = global read "Global 1.vi" "토닉 카메라 값"() -> (w1048:string)
                n806 = invoke class="PrimaryInterfaceScript" method="Send"(reference=w1046, "script"=w1048) -> (reference out=w1045:refnum<k24>)  [unwired: 2 in, 3 out]
                n807 = Wait (ms)(milliseconds to wait=u32 8000) -> ()  [unwired: 1 out]
              }
              frame #26 {
                n808 = global write "Global 1.vi" "그리퍼 닫힘"(TRUE ("그리퍼 열림")) -> ()
                n809 = Wait (ms)(milliseconds to wait=u32 300) -> ()  [unwired: 1 out]
              }
              frame #27 {
                n810 = global write "Global 1.vi" "그리퍼 닫힘"(FALSE ("그리퍼 열림")) -> ()
                n811 = Wait (ms)(milliseconds to wait=u32 3000) -> ()  [unwired: 1 out]
              }
              frame #28 {
                # "토닉 들어올리기"
                n812 = global read "Global 1.vi" "토닉 드는 자세"() -> (w1058:string)
                n813 = invoke class="PrimaryInterfaceScript" method="Send"(reference=w1056, "script"=w1058) -> (reference out=w1055:refnum<k24>)  [unwired: 2 in, 3 out]
                n814 = Wait (ms)(milliseconds to wait=u32 5000) -> ()  [unwired: 1 out]
              }
              frame #29 {
                # "토닉 살짝 빼기"
                n815 = global read "Global 1.vi" "토닉 빼는 자세"() -> (w1062:string)
                n816 = invoke class="PrimaryInterfaceScript" method="Send"(reference=w1060, "script"=w1062) -> (reference out=w1059:refnum<k24>)  [unwired: 2 in, 3 out]
                n817 = Wait (ms)(milliseconds to wait=u32 7000) -> ()  [unwired: 1 out]
              }
              frame #30 {
                # "술잔으로 이동"
                n818 = global read "Global 1.vi" "술잔 위로 가는 자세 2"() -> (w1066:string)
                n819 = invoke class="PrimaryInterfaceScript" method="Send"(reference=w1064, "script"=w1066) -> (reference out=w1063:refnum<k24>)  [unwired: 2 in, 3 out]
                n820 = Wait (ms)(milliseconds to wait=u32 12000) -> ()  [unwired: 1 out]
              }
              frame #31 {
                # "술잔에 따르기"
                n821 = global read "Global 1.vi" "술 따르는 자세 2"() -> (w1070:string)
                n822 = invoke class="PrimaryInterfaceScript" method="Send"(reference=w1068, "script"=w1070) -> (reference out=w1067:refnum<k24>)  [unwired: 2 in, 3 out]
                n823 = Wait (ms)(milliseconds to wait=u32 13000) -> ()  [unwired: 1 out]
              }
              frame #32 {
                # "술따르기 중단"
                n824 = global read "Global 1.vi" "술잔 위로 가는 자세 2"() -> (w1074:string)
                n825 = invoke class="PrimaryInterfaceScript" method="Send"(reference=w1072, "script"=w1074) -> (reference out=w1071:refnum<k24>)  [unwired: 2 in, 3 out]
                n826 = Wait (ms)(milliseconds to wait=u32 5000) -> ()  [unwired: 1 out]
              }
              frame #33 {
                # "토닉 뻇던 자세로 복귀"
                n827 = global read "Global 1.vi" "토닉 빼는 자세"() -> (w1077:string)
                n828 = invoke class="PrimaryInterfaceScript" method="Send"(reference=w1076, "script"=w1077) -> (reference out=w1075:refnum<k24>)  [unwired: 2 in, 3 out]
                n829 = Wait (ms)(milliseconds to wait=u32 9000) -> ()  [unwired: 1 out]
              }
              frame #34 {
                # "토닉 내려놓으러 가기"
                n830 = global read "Global 1.vi" "토닉 드는 자세"() -> (w1082:string)
                n831 = invoke class="PrimaryInterfaceScript" method="Send"(reference=w1080, "script"=w1082) -> (reference out=w1079:refnum<k24>)  [unwired: 2 in, 3 out]
                n832 = Wait (ms)(milliseconds to wait=u32 7000) -> ()  [unwired: 1 out]
              }
              frame #35 {
                # "토닉 내려놓기"
                n833 = global read "Global 1.vi" "토닉 가는자세"() -> (w1086:string)
                n834 = invoke class="PrimaryInterfaceScript" method="Send"(reference=w1084, "script"=w1086) -> (reference out=w1083:refnum<k24>)  [unwired: 2 in, 3 out]
                n835 = Wait (ms)(milliseconds to wait=u32 5000) -> ()  [unwired: 1 out]
              }
              frame #36 {
                # "그리퍼 열기"
                n836 = global write "Global 1.vi" "그리퍼 열림"(TRUE ("그리퍼 열림")) -> ()
                n837 = Wait (ms)(milliseconds to wait=u32 300) -> ()  [unwired: 1 out]
              }
              frame #37 {
                n838 = global write "Global 1.vi" "그리퍼 열림"(FALSE ("그리퍼 열림")) -> ()
                n839 = Wait (ms)(milliseconds to wait=u32 3000) -> ()  [unwired: 1 out]
              }
              frame #38 {
                # "토닉 뻇던 자세로 복귀"
                n840 = global read "Global 1.vi" "토닉 빼는 자세"() -> (w1095:string)
                n841 = invoke class="PrimaryInterfaceScript" method="Send"(reference=w1094, "script"=w1095) -> (reference out=w1093:refnum<k24>)  [unwired: 2 in, 3 out]
                n842 = Wait (ms)(milliseconds to wait=u32 5000) -> ()  [unwired: 1 out]
              }
              frame #39 {
                # "초기자세"
                n843 = global read "Global 1.vi" "1자로 서는 자세"() -> (w1099:string)
                n844 = invoke class="PrimaryInterfaceScript" method="Send"(reference=w1097, "script"=w1099) -> ()  [unwired: 2 in, 4 out]
                n845 = Wait (ms)(milliseconds to wait=u32 15000) -> ()  [unwired: 1 out]
              }
              frame #40 {
                n846 = global write "Global 1.vi" "그리퍼 닫힘"(TRUE ("그리퍼 열림")) -> ()
                n847 = Wait (ms)(milliseconds to wait=u32 300) -> ()  [unwired: 1 out]
              }
              frame #41 {
                w1102 = ""
                # "그리퍼의 앙다문 일자 입"
                n848 = global write "Global 1.vi" "그리퍼 닫힘"(FALSE ("그리퍼 열림")) -> ()
                n849 = Wait (ms)(milliseconds to wait=u32 3000) -> ()  [unwired: 1 out]
                n850 = global write "Global 1.vi" "잭다니엘 카메라 값"(w1102) -> ()
                n851 = global write "Global 1.vi" "콜라 카메라 값"(w1102) -> ()
                n852 = global write "Global 1.vi" "토닉 카메라 값"(w1102) -> ()
                n853 = global write "Global 1.vi" "짐빔 카메라 값"(w1102) -> ()
              }
            }
          }
          frame 5 {
            # "multi order"
          }
          frame 6 {
            # "multi order"
          }
          frame 7 {
            # "multi order"
          }
        }
        n854 = case shown="True" "Send script" {
          tunnel: w50 -> [_ w1111]
          frame False {
          }
          frame True {
            n855 = flat-sequence {
              tunnel: w1111 -> [w1113]
              frame #0 {
                n856 = invoke class="PrimaryInterfaceScript" method="Send"(reference=w1113, "script"="Script to execute") -> ()  [unwired: 2 in, 4 out]
              }
            }
          }
        }
        n857 = case shown="True" "Move to Zero position" {
          tunnel: w50 -> [_ w1108]
          frame False {
          }
          frame True {
            n858 = flat-sequence {
              tunnel: w1108 -> [w1110]
              frame #0 {
                n859 = invoke class="PrimaryInterfaceScript" method="Send"(reference=w1110, "script"="movej([3.1412,-1.5708,0,-1.5708,3.1412,5.8904], a=0.5, v=0.25, t=0, r=0)") -> ()  [unwired: 2 in, 4 out]
              }
            }
          }
        }
        n860 = case shown="True" "Move to particular posture" {
          tunnel: w50 -> [_ w1105]
          frame False {
          }
          frame True {
            n861 = flat-sequence {
              tunnel: w1105 -> [w1107]
              frame #0 {
                n862 = invoke class="PrimaryInterfaceScript" method="Send"(reference=w1107, "script"="movej([-1.5,-1.5,-2,-0.5,1.8,0], a=1.4, v=1.05, t=0, r=0)") -> ()  [unwired: 2 in, 4 out]
              }
            }
          }
        }
        n863 = property class="PrimaryInterfaceClientInternal"(reference=w49) -> ("RobotModeData"=w62:refnum<k24>)  [unwired: 1 in, 2 out]
        n864 = property class="PrimaryInterfaceClientInternal"(reference=w49) -> ("CartesianInfo"=w48:refnum<k24>)  [unwired: 1 in, 2 out]
        n865 = property class="RobotModeDataPackageEventArgs"(reference=w62) -> ("RobotPowerOn"=→"Powered on":bool)  [unwired: 1 in, 2 out]
        n866 = constructor class="SocketCommunicationServer"() -> (reference out=w58:refnum<k24>)  [unwired: 3 in, 2 out]
        n867 = property class="SocketCommunicationServer"(reference=w58) -> ("Enabled"=→"Enabled":bool)  [unwired: 1 in, 2 out]
        n868 = property class="SocketCommunicationServer"(reference=w58) -> ("Port"=→"Port":i32)  [unwired: 1 in, 2 out]
        n869 = property class="CartesianInfoPackageEventArgs"(reference=w48) -> ("Y"=→"Y":dbl)  [unwired: 1 in, 2 out]
        n870 = property class="CartesianInfoPackageEventArgs"(reference=w48) -> ("Ry"=→"Ry":dbl)  [unwired: 1 in, 2 out]
        n871 = property class="CartesianInfoPackageEventArgs"(reference=w48) -> ("Z"=→"Z":dbl)  [unwired: 1 in, 2 out]
        n872 = property class="CartesianInfoPackageEventArgs"(reference=w48) -> ("Rz"=→"Rz":dbl)  [unwired: 1 in, 2 out]
        n873 = property class="CartesianInfoPackageEventArgs"(reference=w48) -> ("X"=→"X":dbl)  [unwired: 1 in, 2 out]
        n874 = property class="CartesianInfoPackageEventArgs"(reference=w48) -> ("Rx"=→"Rx":dbl)  [unwired: 1 in, 2 out]
      }
    }
    n875 = property class="UR"(reference=w33) -> ("Dashboard"=w37:refnum<k24>)  [unwired: 1 in, 2 out]
    n876 = case shown="True" "Power off" {
      tunnel: w37 -> [_ w1114]
      frame False {
      }
      frame True {
        n877 = flat-sequence {
          tunnel: w1114 -> [w1115]
          frame #0 {
            n878 = invoke class="DashboardClientInternal" method="PowerOff"(reference=w1115) -> ()  [unwired: 2 in, 3 out]
          }
        }
      }
    }
    n879 = case shown="True" "Power on\nRelease brake" {
      tunnel: w37 -> [_ w1116]
      frame False {
      }
      frame True {
        n880 = flat-sequence {
          tunnel: w1116 -> [w1118]
          frame #0 {
            n881 = invoke class="DashboardClientInternal" method="PowerOn"(reference=w1118) -> (reference out=w1117:refnum<k24>)  [unwired: 2 in, 2 out]
            n882 = invoke class="DashboardClientInternal" method="ReleaseBrake"(reference=w1117) -> ()  [unwired: 2 in, 3 out]
          }
        }
      }
    }
  }
  n883 = invoke class="UR" method="RegisterLicense"(reference=w27, "licensee"="your company name", "key"="") -> (reference out=w29:refnum<k24>)  [unwired: 2 in, 4 out]
  n884 = control-ref of="Script to execute"() -> (w26:refnum<vi>)
  n885 = property class="Str"(reference=w26, "Value"="movej([-1.5,-1.5,-2,-0.5,1.8,0], a=1.4, v=1.05, t=0, r=0)") -> ()  [unwired: 1 in, 2 out]
  n886 = property class="UR"(reference=w29) -> ("LicenseInfo"=w28:refnum<k24>)  [unwired: 1 in, 2 out]
  n887 = invoke class="LicenseInfo" method="ToString"(reference=w28) -> ("ToString"=→"License state":string)  [unwired: 2 in, 2 out]
  n888 = while {
    stop <- "stop" stop-if-true
    n889 = global read "Global 1.vi" "TCP 스위치"() -> (w1124:bool)
    n890 = case shown="True" w1124 {
      frame False {
        w1126 = "0"
        n891 = global write "Global 1.vi" "지호씨가 보낸 총 좌표"(w1126) -> ()
        n892 = global write "Global 1.vi" "RY_havetogo"(w1126) -> ()
        n893 = global write "Global 1.vi" "RZ_havetogo"(w1126) -> ()
        n894 = global write "Global 1.vi" "RX_havetogo"(w1126) -> ()
        n895 = global write "Global 1.vi" "Y_havetogo"(w1126) -> ()
        n896 = global write "Global 1.vi" "Z_havetogo"(w1126) -> ()
        n897 = global write "Global 1.vi" "X_havetogo"(w1126) -> ()
        n898 = global write "Global 1.vi" "RY_부호"(w1126) -> ()
        n899 = global write "Global 1.vi" "RZ_부호"(w1126) -> ()
        n900 = global write "Global 1.vi" "RX_부호"(w1126) -> ()
        n901 = global write "Global 1.vi" "Y_부호"(w1126) -> ()
        n902 = global write "Global 1.vi" "Z_부호"(w1126) -> ()
        n903 = global write "Global 1.vi" "X_부호"(w1126) -> ()
      }
      frame True {
        w1163 = 4 ("length (rest)")
        n904 = global read "Global 1.vi" "몇번 병을 볼것인가"() -> (w1154:string)
        n905 = TCP Open Connection(address="192.168.112.18", remote port or service name=u16 8089) -> (connection ID=w1158:refnum<k5>, error out=w1157:errorcluster)  [unwired: 3 in]
        n906 = TCP Write(connection ID=w1158, data in=w1154, error in (no error)=w1157) -> (connection ID out=w1156:refnum<k5>, error out=w1155:errorcluster)  [unwired: 1 in, 1 out]
        n907 = TCP Read(connection ID=w1156, bytes to read=30, error in (no error)=w1155, 7:T1."Buffered" ("mode (standard)")) -> (connection ID out=w1167:refnum<k5>, data out=w1127:string, error out=w1166:errorcluster)  [unwired: 1 in]
        n908 = String Subset(string=w1127, offset (0)=11, length (rest)=w1163) -> (substring=w1145:string)
        n909 = String Subset(string=w1127, offset (0)=16, length (rest)=w1163) -> (substring=w1144:string)
        n910 = String Subset(string=w1127, offset (0)=6, length (rest)=w1163) -> (substring=w1146:string)
        n911 = String Subset(string=w1127, offset (0)=1, length (rest)=w1163) -> (substring=w1147:string)
        n912 = global write "Global 1.vi" "X_havetogo"(w1147) -> ()
        n913 = global write "Global 1.vi" "Z_havetogo"(w1145) -> ()
        n914 = global write "Global 1.vi" "RX_havetogo"(w1144) -> ()
        n915 = global write "Global 1.vi" "Y_havetogo"(w1146) -> ()
        n916 = String Subset(string=w1127, offset (0)=26, length (rest)=w1163) -> (substring=w1142:string)
        n917 = String Subset(string=w1127, offset (0)=21, length (rest)=w1163) -> (substring=w1143:string)
        n918 = global write "Global 1.vi" "지호씨가 보낸 총 좌표"(w1127) -> ()
        n919 = String Subset(string=w1127, offset (0)=20, length (rest)=1 ("length (rest)")) -> (substring=w1140:string)
        n920 = String Subset(string=w1127, offset (0)=15, length (rest)=1 ("length (rest)")) -> (substring=w1141:string)
        n921 = String Subset(string=w1127, offset (0)=25, length (rest)=1 ("length (rest)")) -> (substring=w1139:string)
        n922 = global write "Global 1.vi" "RY_havetogo"(w1143) -> ()
        n923 = TCP Close Connection(connection ID=w1167, error in (no error)=w1166) -> ()  [unwired: 1 in, 2 out]
        n924 = global write "Global 1.vi" "RZ_havetogo"(w1142) -> ()
        n925 = global write "Global 1.vi" "RY_부호"(w1140) -> ()
        n926 = global write "Global 1.vi" "RX_부호"(w1141) -> ()
        n927 = global write "Global 1.vi" "RZ_부호"(w1139) -> ()
        n928 = String Subset(string=w1127, offset (0)=0, length (rest)=1 ("length (rest)")) -> (substring=w1136:string)
        n929 = String Subset(string=w1127, offset (0)=5, length (rest)=1 ("length (rest)")) -> (substring=w1133:string)
        n930 = String Subset(string=w1127, offset (0)=10, length (rest)=1 ("length (rest)")) -> (substring=w1130:string)
        n931 = global write "Global 1.vi" "X_부호"(w1136) -> ()
        n932 = global write "Global 1.vi" "Y_부호"(w1133) -> ()
        n933 = global write "Global 1.vi" "Z_부호"(w1130) -> ()
      }
    }
    n934 = Wait Until Next ms Multiple(millisecond multiple=u32 100) -> ()  [unwired: 1 out]
  }
